vi "Set all to no debugging.vi"() -> ()   [LabVIEW 2013]
doc: "This .vi searches all .vi's in memory and returns a list sorted by the amount memory they are using. This .vi is helpful to find .vis that have stored large amounts of data on the diagram or in the default values."
panel:
  in  "Debug?":bool
  out "total # of .vis":i32=1555
  out "Array":T1(array[cluster])=[{"Boolean"=FALSE, "Boolean 2"=FALSE, "Name"="Quartz MAIN.vi", "Boolean 3"=FALSE}, {"Boolean"=FALSE, "Boolean 2"=FALSE, "Name"="PI Open Interface of one system.vi", "Boolean 3"=FALSE}, {"Boolean"=FALSE, "Boolean 2"=FALSE, "Name"="GCSTranslator DLL Functions.vi", "Boolean 3"=FALSE}, {"Boolean"=FALSE, "Boolean 2"=FALSE, "Name"="HHMI - Zernike GUI.vi", "Boolean 3"=FALSE}, {"Boolean"=FALSE, "Boolean 2"=FALSE, "Name"="Quartz SLM utility.vi", "Boolean 3"=FALSE}, {"Boolean"=FALSE, "Boolean 2"=FALSE, "Name"="HHMI - AO mask definitions.vi", "Boolean 3"=FALSE}, {"Boolean"=FALSE, "Boolean 2"=FALSE, "Name"="Quartz Reviewer.vi", "Boolean 3"=FALSE}, {"Boolean"=FALSE, "Boolean 2"=FALSE, "Name"="C867_Configuration_Setup.vi", "Boolean 3"=FALSE}, {"Boolean"=FALSE, "Boolean 2"=FALSE, "Name"="HHMI - AO Scan Independent mode.vi", "Boolean 3"=FALSE}, {"Boolean"=FALSE, "Boolean 2"=FALSE, "Name"="HHMI - Pick XYlineZ GUI.vi", "Boolean 3"=FALSE}, {"Boolean"=FALSE, "Boolean 2"=FALSE, "Name"="HHMI - Optimize SLM angles and phases simplified inverse.vi", "Boolean 3"=FALSE}, {"Boolean"=FALSE, "Boolean 2"=FALSE, "Name"="HHMI - AO Overlap mode.vi", "Boolean 3"=FALSE}, {"Boolean"=FALSE, "Boolean 2"=FALSE, "Name"="HHMI - AO Scan Masks mode.vi", "Boolean 3"=FALSE}, {"Boolean"=FALSE, "Boolean 2"=FALSE, "Name"="HHMI - SLM Control Module.vi", "Boolean 3"=FALSE}, {"Boolean"=FALSE, "Boolean 2"=FALSE, "Name"="General wait for movement to stop.vi", "Boolean 3"=FALSE}, {"Boolean"=FALSE, "Boolean 2"=FALSE, "Name"="HHMI - Optimize SLM angles and phases for Masks.vi", "Boolean 3"=FALSE}, {"Boolean"=FALSE, "Boolean 2"=FALSE, "Name"="Select DaisyChain device.vi", "Boolean 3"=FALSE}, {"Boolean"=FALSE, "Boolean 2"=FALSE, "Name"="HHMI - AO Scan Inverse mode.vi", "Boolean 3"=FALSE}, {"Boolean"=FALSE, "Boolean 2"=FALSE, "Name"="HHMI - Optimize SLM angles independent montage.vi", "Boolean 3"=FALSE}, {"Boolean"=FALSE, "Boolean 2"=FALSE, "Name"="Select USB device.vi", "Boolean 3"=FALSE}, {"Boolean"=FALSE, "Boolean 2"=FALSE, "Name"="32 bit tiff reader.lvlib:Load Flattened 32bit float Image from Tiff.vi", "Boolean 3"=FALSE}, {"Boolean"=FALSE, "Boolean 2"=FALSE, "Name"="HHMI - Motion GUI.vi", "Boolean 3"=FALSE}, {"Boolean"=FALSE, "Boolean 2"=FALSE, "Name"="HHMI - Align to SLM center calibrate BR image shift Scan module.vi", "Boolean 3"=FALSE}, {"Boolean"=FALSE, "Boolean 2"=FALSE, "Name"="HHMI - Optimize SLM angles simplified inverse.vi", "Boolean 3"=FALSE}, {"Boolean"=FALSE, "Boolean 2"=FALSE, "Name"="HHMI - AO Power Manager.vi", "Boolean 3"=FALSE}, {"Boolean"=FALSE, "Boolean 2"=FALSE, "Name"="HHMI - Optimize SLM phases independent.vi", "Boolean 3"=FALSE}, {"Boolean"=FALSE, "Boolean 2"=FALSE, "Name"="su10x Get Filter Wheel Status.vi", "Boolean 3"=FALSE}, {"Boolean"=FALSE, "Boolean 2"=FALSE, "Name"="PI Receive String.vi", "Boolean 3"=FALSE}, {"Boolean"=FALSE, "Boolean 2"=FALSE, "Name"="HHMI - Optimize SLM angles Masks.vi", "Boolean 3"=FALSE}, {"Boolean"=FALSE, "Boolean 2"=FALSE, "Name"="HHMI - Optimize SLM phase of 1 mask.vi", "Boolean 3"=FALSE}, {"Boolean"=FALSE, "Boolean 2"=FALSE, "Name"="HHMI - Align to each SLM subregion Scan module.vi", "Boolean 3"=FALSE}, {"Boolean"=FALSE, "Boolean 2"=FALSE, "Name"="HHMI - Optimize SLM phase of 1 subregion independent.vi", "Boolean 3"=FALSE}, {"Boolean"=FALSE, "Boolean 2"=FALSE, "Name"="HHMI - PI laser motion module.vi", "Boolean 3"=FALSE}, {"Boolean"=FALSE, "Boolean 2"=FALSE, "Name"="HHMI - Optimize SLM angles Overlap.vi", "Boolean 3"=FALSE}, {"Boolean"=FALSE, "Boolean 2"=FALSE, "Name"="Adjust Laser positioner Calibration GUI.vi", "Boolean 3"=FALSE}, {"Boolean"=FALSE, "Boolean 2"=FALSE, "Name"="HHMI - Optimize SLM angles independent.vi", "Boolean 3"=FALSE}, {"Boolean"=FALSE, "Boolean 2"=FALSE, "Name"="HHMI - Optimize SLM phase of 1 subsubregion inverse.vi", "Boolean 3"=FALSE}, {"Boolean"=FALSE, "Boolean 2"=FALSE, "Name"="HHMI - Optimize SLM angles and phases for Overlap.vi", "Boolean 3"=FALSE}, {"Boolean"=FALSE, "Boolean 2"=FALSE, "Name"="Assign values from string to axes.vi", "Boolean 3"=FALSE}, {"Boolean"=FALSE, "Boolean 2"=FALSE, "Name"="HHMI - Subregion On Scan module.vi", "Boolean 3"=FALSE}, {"Boolean"=FALSE, "Boolean 2"=FALSE, "Name"="HHMI - Working images - create and keep reference.vi", "Boolean 3"=FALSE}, {"Boolean"=FALSE, "Boolean 2"=FALSE, "Name"="HHMI - Joystick control loop.vi", "Boolean 3"=FALSE}, {"Boolean"=FALSE, "Boolean 2"=FALSE, "Name"="HHMI - Subregion Off Scan module.vi", "Boolean 3"=FALSE}, {"Boolean"=FALSE, "Boolean 2"=FALSE, "Name"="HHMI - Calc Single X Line Ramp.vi", "Boolean 3"=FALSE}, {"Boolean"=FALSE, "Boolean 2"=FALSE, "Name"="HHMI - Linescan Scan module.vi", "Boolean 3"=FALSE}, {"Boolean"=FALSE, "Boolean 2"=FALSE, "Name"="HHMI - Analysis Table module.vi", "Boolean 3"=FALSE}, {"Boolean"=FALSE, "Boolean 2"=FALSE, "Name"="HHMI - Retrieve All Settings from globals.vi", "Boolean 3"=FALSE}, {"Boolean"=FALSE, "Boolean 2"=FALSE, "Name"="HHMI - Center laser along one axis module.vi", "Boolean 3"=FALSE}, {"Boolean"=FALSE, "Boolean 2"=FALSE, "Name"="HHMI - Center laser to on subregions module.vi", "Boolean 3"=FALSE}, {"Boolean"=FALSE, "Boolean 2"=FALSE, "Name"="SO Beam expander.lvlib:SO - BE Controller used now for calibration only.vi", "Boolean 3"=FALSE}, {"Boolean"=FALSE, "Boolean 2"=FALSE, "Name"="HHMI - Beam size control module.vi", "Boolean 3"=FALSE}, {"Boolean"=FALSE, "Boolean 2"=FALSE, "Name"="HHMI - Z Stack Scan module.vi", "Boolean 3"=FALSE}, {"Boolean"=FALSE, "Boolean 2"=FALSE, "Name"="HHMI - Optimize SLM phases for Masks.vi", "Boolean 3"=FALSE}, {"Boolean"=FALSE, "Boolean 2"=FALSE, "Name"="HHMI - Global ramp generate subregion offsets.vi", "Boolean 3"=FALSE}, {"Boolean"=FALSE, "Boolean 2"=FALSE, "Name"="HHMI - Locate blob.vi", "Boolean 3"=FALSE}, {"Boolean"=FALSE, "Boolean 2"=FALSE, "Name"="PI Send String.vi", "Boolean 3"=FALSE}, {"Boolean"=FALSE, "Boolean 2"=FALSE, "Name"="HHMI - Increase OL subregion resolution and extend planes to border.vi", "Boolean 3"=FALSE}, {"Boolean"=FALSE, "Boolean 2"=FALSE, "Name"="HHMI - PI beam reducer module.vi", "Boolean 3"=FALSE}, {"Boolean"=FALSE, "Boolean 2"=FALSE, "Name"="HHMI - Align to SLM active area Scan module.vi", "Boolean 3"=FALSE}, {"Boolean"=FALSE, "Boolean 2"=FALSE, "Name"="HHMI - Wait for scan to finish.vi", "Boolean 3"=FALSE}, {"Boolean"=FALSE, "Boolean 2"=FALSE, "Name"="HHMI - Configure for scan.vi", "Boolean 3"=FALSE}, {"Boolean"=FALSE, "Boolean 2"=FALSE, "Name"="HHMI - Optimize SLM phase simplified inverse.vi", "Boolean 3"=FALSE}, {"Boolean"=FALSE, "Boolean 2"=FALSE, "Name"="Adjust BR Calibration GUI.vi", "Boolean 3"=FALSE}, {"Boolean"=FALSE, "Boolean 2"=FALSE, "Name"="HHMI - Adjust power up or down based on current signal.vi", "Boolean 3"=FALSE}, {"Boolean"=FALSE, "Boolean 2"=FALSE, "Name"="Assign booleans from string to axes.vi", "Boolean 3"=FALSE}, {"Boolean"=FALSE, "Boolean 2"=FALSE, "Name"="HHMI - Generate Waveform.vi", "Boolean 3"=FALSE}, {"Boolean"=FALSE, "Boolean 2"=FALSE, "Name"="HHMI - Stage 1 optimized beamlet settings storage global.vi", "Boolean 3"=FALSE}, {"Boolean"=FALSE, "Boolean 2"=FALSE, "Name"="HHMI - Optimized Beamlet settings storage global.vi", "Boolean 3"=FALSE}, {"Boolean"=FALSE, "Boolean 2"=FALSE, "Name"="Alignment GUI.vi", "Boolean 3"=FALSE}, {"Boolean"=FALSE, "Boolean 2"=FALSE, "Name"="HHMI - Scan.vi", "Boolean 3"=FALSE}, {"Boolean"=FALSE, "Boolean 2"=FALSE, "Name"="HHMI - Convert one channel to Pixels.vi", "Boolean 3"=FALSE}, {"Boolean"=FALSE, "Boolean 2"=FALSE, "Name"="HHMI - Select a coordinate GUI.vi", "Boolean 3"=FALSE}, {"Boolean"=FALSE, "Boolean 2"=FALSE, "Name"="HHMI - Magnify and Center waveform on phase signal area.vi", "Boolean 3"=FALSE}, {"Boolean"=FALSE, "Boolean 2"=FALSE, "Name"="HHMI - Shift waveforms by galvo delay.vi", "Boolean 3"=FALSE}, {"Boolean"=FALSE, "Boolean 2"=FALSE, "Name"="HHMI - Generate 1 Frame Sine.vi", "Boolean 3"=FALSE}, {"Boolean"=FALSE, "Boolean 2"=FALSE, "Name"="HHMI - Generate 1 Frame Ramp.vi", "Boolean 3"=FALSE}, {"Boolean"=FALSE, "Boolean 2"=FALSE, "Name"="HHMI - XY Galvo control module.vi", "Boolean 3"=FALSE}, {"Boolean"=FALSE, "Boolean 2"=FALSE, "Name"="HHMI - Generate subdivided subsubregions.vi", "Boolean 3"=FALSE}, {"Boolean"=FALSE, "Boolean 2"=FALSE, "Name"="HHMI - Lev Mar.vi", "Boolean 3"=FALSE}, {"Boolean"=FALSE, "Boolean 2"=FALSE, "Name"="HHMI - AO Dev3 control module.vi", "Boolean 3"=FALSE}, {"Boolean"=FALSE, "Boolean 2"=FALSE, "Name"="HHMI - Z Pockel control module.vi", "Boolean 3"=FALSE}, {"Boolean"=FALSE, "Boolean 2"=FALSE, "Name"="HHMI - XY Continuous Scan module.vi", "Boolean 3"=FALSE}, {"Boolean"=FALSE, "Boolean 2"=FALSE, "Name"="HHMI - XY Single Scan module.vi", "Boolean 3"=FALSE}, {"Boolean"=FALSE, "Boolean 2"=FALSE, "Name"="HHMI - Dynamically launch Pick XYlineZ GUI.vi", "Boolean 3"=FALSE}, {"Boolean"=FALSE, "Boolean 2"=FALSE, "Name"="HHMI - Initialize for AO Overlap Scan.vi", "Boolean 3"=FALSE}, {"Boolean"=FALSE, "Boolean 2"=FALSE, "Name"="HHMI - Is a new Background scan needed for this waveform config.vi", "Boolean 3"=FALSE}, {"Boolean"=FALSE, "Boolean 2"=FALSE, "Name"="HHMI - Generate 1 Line Sine.vi", "Boolean 3"=FALSE}, {"Boolean"=FALSE, "Boolean 2"=FALSE, "Name"="HHMI - Calc Single Frame Ramp Waveform.vi", "Boolean 3"=FALSE}, {"Boolean"=FALSE, "Boolean 2"=FALSE, "Name"="HHMI - Optimized Beamlet settings for Pre-Angle and Pre-Phase storage global.vi", "Boolean 3"=FALSE}, {"Boolean"=FALSE, "Boolean 2"=FALSE, "Name"="HHMI - Beam reducer in scan and store COM as ref.vi", "Boolean 3"=FALSE}, {"Boolean"=FALSE, "Boolean 2"=FALSE, "Name"="HHMI - ReadWrite Analysis Info.vi", "Boolean 3"=FALSE}, {"Boolean"=FALSE, "Boolean 2"=FALSE, "Name"="HHMI - Z stack settings functional global.vi", "Boolean 3"=FALSE}, {"Boolean"=FALSE, "Boolean 2"=FALSE, "Name"="HHMI - AO Scan wrapper.vi", "Boolean 3"=FALSE}, {"Boolean"=FALSE, "Boolean 2"=FALSE, "Name"="HHMI - Generate 1 Line Ramp.vi", "Boolean 3"=FALSE}, {"Boolean"=FALSE, "Boolean 2"=FALSE, "Name"="HHMI - Turn on one subregion, one mask, or one overlap region on_Also scan if no BR is used.vi", "Boolean 3"=FALSE}, {"Boolean"=FALSE, "Boolean 2"=FALSE, "Name"="HHMI - Fit Phase with Zernike modes using nonlinear fit 1 iteration.vi", "Boolean 3"=FALSE}, {"Boolean"=FALSE, "Boolean 2"=FALSE, "Name"="HHMI - PMT and Integrator Acquisition control module.vi", "Boolean 3"=FALSE}, {"Boolean"=FALSE, "Boolean 2"=FALSE, "Name"="su10x Get Filter Wheel Configuration.vi", "Boolean 3"=FALSE}, {"Boolean"=FALSE, "Boolean 2"=FALSE, "Name"="HHMI - Initialize for Independent AO Scan.vi", "Boolean 3"=FALSE}, {"Boolean"=FALSE, "Boolean 2"=FALSE, "Name"="HHMI - Image Correlation module.vi", "Boolean 3"=FALSE}, {"Boolean"=FALSE, "Boolean 2"=FALSE, "Name"="Joystick controller.vi", "Boolean 3"=FALSE}, {"Boolean"=FALSE, "Boolean 2"=FALSE, "Name"="HHMI - Extend 2D subregion array with one element border.vi", "Boolean 3"=FALSE}, {"Boolean"=FALSE, "Boolean 2"=FALSE, "Name"="HHMI - Initialize for AO Mask Scan.vi", "Boolean 3"=FALSE}, {"Boolean"=FALSE, "Boolean 2"=FALSE, "Name"="HHMI - Background image storage module.vi", "Boolean 3"=FALSE}, {"Boolean"=FALSE, "Boolean 2"=FALSE, "Name"="Cut out additional spaces.vi", "Boolean 3"=FALSE}, {"Boolean"=FALSE, "Boolean 2"=FALSE, "Name"="HHMI - Unwrap Phase.vi", "Boolean 3"=FALSE}, {"Boolean"=FALSE, "Boolean 2"=FALSE, "Name"="HHMI - Send image to logger loop.vi", "Boolean 3"=FALSE}, {"Boolean"=FALSE, "Boolean 2"=FALSE, "Name"="HHMI - Calibrated XY image shift due to beam expander functional global.vi", "Boolean 3"=FALSE}, {"Boolean"=FALSE, "Boolean 2"=FALSE, "Name"="HHMI - Phase Signal storage global.vi", "Boolean 3"=FALSE}, {"Boolean"=FALSE, "Boolean 2"=FALSE, "Name"="HHMI - Convert between Settings cluster and flattenned string.vi", "Boolean 3"=FALSE}, {"Boolean"=FALSE, "Boolean 2"=FALSE, "Name"="HHMI - Optimize SLM phases via wavefront reconstruction.vi", "Boolean 3"=FALSE}, {"Boolean"=FALSE, "Boolean 2"=FALSE, "Name"="HHMI - Goto XYZ.vi", "Boolean 3"=FALSE}, {"Boolean"=FALSE, "Boolean 2"=FALSE, "Name"="HHMI - Cal Zernike Mode.vi", "Boolean 3"=FALSE}, {"Boolean"=FALSE, "Boolean 2"=FALSE, "Name"="Adjust waveform for montage.vi", "Boolean 3"=FALSE}, {"Boolean"=FALSE, "Boolean 2"=FALSE, "Name"="HHMI - Generate Waveform Sine.vi", "Boolean 3"=FALSE}, {"Boolean"=FALSE, "Boolean 2"=FALSE, "Name"="HHMI - Generate Waveform Ramp.vi", "Boolean 3"=FALSE}, {"Boolean"=FALSE, "Boolean 2"=FALSE, "Name"="HHMI - Process image for COM calc.vi", "Boolean 3"=FALSE}, {"Boolean"=FALSE, "Boolean 2"=FALSE, "Name"="HHMI - XY Position and Electrode Acquisition control module.vi", "Boolean 3"=FALSE}, {"Boolean"=FALSE, "Boolean 2"=FALSE, "Name"="Interpolate 2D uneven arrays full calc.vi", "Boolean 3"=FALSE}, {"Boolean"=FALSE, "Boolean 2"=FALSE, "Name"="HHMI - Z elevator motion module.vi", "Boolean 3"=FALSE}, {"Boolean"=FALSE, "Boolean 2"=FALSE, "Name"="HHMI - Scale Image.vi", "Boolean 3"=FALSE}, {"Boolean"=FALSE, "Boolean 2"=FALSE, "Name"="HHMI - Alignment Scan wrapper.vi", "Boolean 3"=FALSE}, {"Boolean"=FALSE, "Boolean 2"=FALSE, "Name"="HHMI - Pockel PD Acquisition control module.vi", "Boolean 3"=FALSE}, {"Boolean"=FALSE, "Boolean 2"=FALSE, "Name"="HHMI - Take Ref scan or scans with one mask on.vi", "Boolean 3"=FALSE}, {"Boolean"=FALSE, "Boolean 2"=FALSE, "Name"="HHMI - Take Ref scan or scans with one overlap region on.vi", "Boolean 3"=FALSE}, {"Boolean"=FALSE, "Boolean 2"=FALSE, "Name"="HHMI - XY table motion module.vi", "Boolean 3"=FALSE}, {"Boolean"=FALSE, "Boolean 2"=FALSE, "Name"="HHMI - Center waveform config at COM coords.vi", "Boolean 3"=FALSE}, {"Boolean"=FALSE, "Boolean 2"=FALSE, "Name"="HHMI - Autoset power functional global.vi", "Boolean 3"=FALSE}, {"Boolean"=FALSE, "Boolean 2"=FALSE, "Name"="HHMI - Fit and Store mask as optimized if improved.vi", "Boolean 3"=FALSE}, {"Boolean"=FALSE, "Boolean 2"=FALSE, "Name"="HHMI - Lookup table for Stage mm to SLM mm functional global.vi", "Boolean 3"=FALSE}, {"Boolean"=FALSE, "Boolean 2"=FALSE, "Name"="Wait for axes to stop.vi", "Boolean 3"=FALSE}, {"Boolean"=FALSE, "Boolean 2"=FALSE, "Name"="HHMI - Scan centered at the COM or Image Correlation user selection.vi", "Boolean 3"=FALSE}, {"Boolean"=FALSE, "Boolean 2"=FALSE, "Name"="HHMI - Subregion Scan wrapper.vi", "Boolean 3"=FALSE}, {"Boolean"=FALSE, "Boolean 2"=FALSE, "Name"="HHMI - Image ROI to XY Parameters.vi", "Boolean 3"=FALSE}, {"Boolean"=FALSE, "Boolean 2"=FALSE, "Name"="HHMI - Extend subregion plane to neighboring subregions.vi", "Boolean 3"=FALSE}, {"Boolean"=FALSE, "Boolean 2"=FALSE, "Name"="HHMI - Check and correct Fast axis params.vi", "Boolean 3"=FALSE}, {"Boolean"=FALSE, "Boolean 2"=FALSE, "Name"="HHMI - Subdivide optimized SLM image.vi", "Boolean 3"=FALSE}, {"Boolean"=FALSE, "Boolean 2"=FALSE, "Name"="HHMI - Prepare for alignment to all SLM regions.vi", "Boolean 3"=FALSE}, {"Boolean"=FALSE, "Boolean 2"=FALSE, "Name"="HHMI - Simulate Scan.vi", "Boolean 3"=FALSE}, {"Boolean"=FALSE, "Boolean 2"=FALSE, "Name"="Wait for hexapod system axes to stop.vi", "Boolean 3"=FALSE}, {"Boolean"=FALSE, "Boolean 2"=FALSE, "Name"="HHMI - Laser Power storage functional global.vi", "Boolean 3"=FALSE}, {"Boolean"=FALSE, "Boolean 2"=FALSE, "Name"="HHMI - All on scan for Masks to accept or reject current mask set.vi", "Boolean 3"=FALSE}, {"Boolean"=FALSE, "Boolean 2"=FALSE, "Name"="HHMI - Calc Single Frame Sine Waveform.vi", "Boolean 3"=FALSE}, {"Boolean"=FALSE, "Boolean 2"=FALSE, "Name"="HHMI - Increase Power Time or Averages to get more Signal.vi", "Boolean 3"=FALSE}, {"Boolean"=FALSE, "Boolean 2"=FALSE, "Name"="HHMI - Calc X Sine Waveform.vi", "Boolean 3"=FALSE}, {"Boolean"=FALSE, "Boolean 2"=FALSE, "Name"="SO Beam expander.lvlib:Gen_7I60_IO.vi", "Boolean 3"=FALSE}, {"Boolean"=FALSE, "Boolean 2"=FALSE, "Name"="HHMI - Generate pattern.vi", "Boolean 3"=FALSE}, {"Boolean"=FALSE, "Boolean 2"=FALSE, "Name"="HHMI - Scan state information to Strings.vi", "Boolean 3"=FALSE}, {"Boolean"=FALSE, "Boolean 2"=FALSE, "Name"="HHMI - Overlap settings to number of duplicate rows and columns.vi", "Boolean 3"=FALSE}, {"Boolean"=FALSE, "Boolean 2"=FALSE, "Name"="HHMI - Background Module.vi", "Boolean 3"=FALSE}, {"Boolean"=FALSE, "Boolean 2"=FALSE, "Name"="HHMI - Overlap wavefront reconstruction storage global.vi", "Boolean 3"=FALSE}, {"Boolean"=FALSE, "Boolean 2"=FALSE, "Name"="Increase image size for montage.vi", "Boolean 3"=FALSE}, {"Boolean"=FALSE, "Boolean 2"=FALSE, "Name"="HHMI - Number of extra counts needed for galvo iteria shift.vi", "Boolean 3"=FALSE}, {"Boolean"=FALSE, "Boolean 2"=FALSE, "Name"="HHMI - SLM Sizes.vi", "Boolean 3"=FALSE}, {"Boolean"=FALSE, "Boolean 2"=FALSE, "Name"="HHMI - Add Signal overlay to image.vi", "Boolean 3"=FALSE}, {"Boolean"=FALSE, "Boolean 2"=FALSE, "Name"="HHMI - Add COM overlay to image.vi", "Boolean 3"=FALSE}, {"Boolean"=FALSE, "Boolean 2"=FALSE, "Name"="SO Beam expander.lvlib:Seek_Home.vi", "Boolean 3"=FALSE}, {"Boolean"=FALSE, "Boolean 2"=FALSE, "Name"="HHMI - Read or write SLM settings.vi", "Boolean 3"=FALSE}, {"Boolean"=FALSE, "Boolean 2"=FALSE, "Name"="HHMI - Check AO rate.vi", "Boolean 3"=FALSE}, {"Boolean"=FALSE, "Boolean 2"=FALSE, "Name"="HHMI - Find Max laser power.vi", "Boolean 3"=FALSE}, {"Boolean"=FALSE, "Boolean 2"=FALSE, "Name"="HHMI - Lock image size.vi", "Boolean 3"=FALSE}, {"Boolean"=FALSE, "Boolean 2"=FALSE, "Name"="Interloop message handler.vi", "Boolean 3"=FALSE}, {"Boolean"=FALSE, "Boolean 2"=FALSE, "Name"="HHMI - Add phase info to table.vi", "Boolean 3"=FALSE}, {"Boolean"=FALSE, "Boolean 2"=FALSE, "Name"="HHMI - Generate Slow axis array for sine.vi", "Boolean 3"=FALSE}, {"Boolean"=FALSE, "Boolean 2"=FALSE, "Name"="HHMI - Pixel Clock control module.vi", "Boolean 3"=FALSE}, {"Boolean"=FALSE, "Boolean 2"=FALSE, "Name"="SO Beam expander.lvlib:Tweak.vi", "Boolean 3"=FALSE}, {"Boolean"=FALSE, "Boolean 2"=FALSE, "Name"="HHMI - Place subregion array into display array.vi", "Boolean 3"=FALSE}, {"Boolean"=FALSE, "Boolean 2"=FALSE, "Name"="HHMI - Image buffer logger.vi", "Boolean 3"=FALSE}, {"Boolean"=FALSE, "Boolean 2"=FALSE, "Name"="SAI?.vi", "Boolean 3"=FALSE}, {"Boolean"=FALSE, "Boolean 2"=FALSE, "Name"="HHMI - Beam reducer shift image in waveform.vi", "Boolean 3"=FALSE}, {"Boolean"=FALSE, "Boolean 2"=FALSE, "Name"="HHMI - Crop SLM pixels to subregions.vi", "Boolean 3"=FALSE}, {"Boolean"=FALSE, "Boolean 2"=FALSE, "Name"="SO Beam expander.lvlib:Read Config INI.vi", "Boolean 3"=FALSE}, {"Boolean"=FALSE, "Boolean 2"=FALSE, "Name"="HHMI - Check Coordinates.vi", "Boolean 3"=FALSE}, {"Boolean"=FALSE, "Boolean 2"=FALSE, "Name"="HHMI - Read write Axis cluster from Waveform.vi", "Boolean 3"=FALSE}, {"Boolean"=FALSE, "Boolean 2"=FALSE, "Name"="HHMI - AO move Beam reducer.vi", "Boolean 3"=FALSE}, {"Boolean"=FALSE, "Boolean 2"=FALSE, "Name"="HHMI - Displacement Data storage global.vi", "Boolean 3"=FALSE}, {"Boolean"=FALSE, "Boolean 2"=FALSE, "Name"="Is DaisyChain open.vi", "Boolean 3"=FALSE}, {"Boolean"=FALSE, "Boolean 2"=FALSE, "Name"="HHMI - Generate Zernike Bar graph.vi", "Boolean 3"=FALSE}, {"Boolean"=FALSE, "Boolean 2"=FALSE, "Name"="HHMI - Calc optimized offset of multiple subregions using neighboring subregions.vi", "Boolean 3"=FALSE}, {"Boolean"=FALSE, "Boolean 2"=FALSE, "Name"="HHMI - Set Reducer and waveform.vi", "Boolean 3"=FALSE}, {"Boolean"=FALSE, "Boolean 2"=FALSE, "Name"="HHMI - Calculate Signal.vi", "Boolean 3"=FALSE}, {"Boolean"=FALSE, "Boolean 2"=FALSE, "Name"="HHMI - Integrator Pulse control module.vi", "Boolean 3"=FALSE}, {"Boolean"=FALSE, "Boolean 2"=FALSE, "Name"="HHMI - Store current settings as initial speed and power.vi", "Boolean 3"=FALSE}, {"Boolean"=FALSE, "Boolean 2"=FALSE, "Name"="HHMI - Overlap settings to number of rows and columns.vi", "Boolean 3"=FALSE}, {"Boolean"=FALSE, "Boolean 2"=FALSE, "Name"="HHMI - Load SLM image from file.vi", "Boolean 3"=FALSE}, {"Boolean"=FALSE, "Boolean 2"=FALSE, "Name"="Interpolate 2D uneven arrays linear fit row by row.vi", "Boolean 3"=FALSE}, {"Boolean"=FALSE, "Boolean 2"=FALSE, "Name"="HHMI - Reset Waveform Configuration to initial power and scan speed.vi", "Boolean 3"=FALSE}, {"Boolean"=FALSE, "Boolean 2"=FALSE, "Name"="HHMI - Is SLM setup for masks.vi", "Boolean 3"=FALSE}, {"Boolean"=FALSE, "Boolean 2"=FALSE, "Name"="HHMI - Generate subregion block from subregion settings.vi", "Boolean 3"=FALSE}, {"Boolean"=FALSE, "Boolean 2"=FALSE, "Name"="HHMI - Set power for 1 mask.vi", "Boolean 3"=FALSE}, {"Boolean"=FALSE, "Boolean 2"=FALSE, "Name"="HHMI - Load Image and Settings from File.vi", "Boolean 3"=FALSE}, {"Boolean"=FALSE, "Boolean 2"=FALSE, "Name"="SO Beam expander.lvlib:Intialize Serial Port.vi", "Boolean 3"=FALSE}, {"Boolean"=FALSE, "Boolean 2"=FALSE, "Name"="HHMI - Prepare for alignment to active SLM regions.vi", "Boolean 3"=FALSE}, {"Boolean"=FALSE, "Boolean 2"=FALSE, "Name"="HHMI - Unwrap Phase down each row of subregions.vi", "Boolean 3"=FALSE}, {"Boolean"=FALSE, "Boolean 2"=FALSE, "Name"="HHMI - Unwrap Phase down each column of subregions.vi", "Boolean 3"=FALSE}, {"Boolean"=FALSE, "Boolean 2"=FALSE, "Name"="HHMI - AO set beam size.vi", "Boolean 3"=FALSE}, {"Boolean"=FALSE, "Boolean 2"=FALSE, "Name"="HHMI - Subregion powers and dwell time functional global.vi", "Boolean 3"=FALSE}, {"Boolean"=FALSE, "Boolean 2"=FALSE, "Name"="HHMI - Digital input output DC control module.vi", "Boolean 3"=FALSE}, {"Boolean"=FALSE, "Boolean 2"=FALSE, "Name"="HHMI - Find ROI.vi", "Boolean 3"=FALSE}, {"Boolean"=FALSE, "Boolean 2"=FALSE, "Name"="HHMI - Sutter filter wheel module.vi", "Boolean 3"=FALSE}, {"Boolean"=FALSE, "Boolean 2"=FALSE, "Name"="Initialize Global1.vi", "Boolean 3"=FALSE}, {"Boolean"=FALSE, "Boolean 2"=FALSE, "Name"="HHMI - Reduce Power to prevent saturation.vi", "Boolean 3"=FALSE}, {"Boolean"=FALSE, "Boolean 2"=FALSE, "Name"="HHMI - Signal vs Motion storage global.vi", "Boolean 3"=FALSE}, {"Boolean"=FALSE, "Boolean 2"=FALSE, "Name"="HHMI - Line Profile.vi", "Boolean 3"=FALSE}, {"Boolean"=FALSE, "Boolean 2"=FALSE, "Name"="su10x Initialize.vi", "Boolean 3"=FALSE}, {"Boolean"=FALSE, "Boolean 2"=FALSE, "Name"="HHMI - Add File image pixels to SLM subregion.vi", "Boolean 3"=FALSE}, {"Boolean"=FALSE, "Boolean 2"=FALSE, "Name"="HHMI - SLM pixels to Laser mm functional global.vi", "Boolean 3"=FALSE}, {"Boolean"=FALSE, "Boolean 2"=FALSE, "Name"="HHMI - Set the previous power and dwell time for a subregion.vi", "Boolean 3"=FALSE}, {"Boolean"=FALSE, "Boolean 2"=FALSE, "Name"="SO Beam expander.lvlib:Move Both.vi", "Boolean 3"=FALSE}, {"Boolean"=FALSE, "Boolean 2"=FALSE, "Name"="HHMI - Move Laser on SLM.vi", "Boolean 3"=FALSE}, {"Boolean"=FALSE, "Boolean 2"=FALSE, "Name"="HHMI - Set power for 1 overlap region.vi", "Boolean 3"=FALSE}, {"Boolean"=FALSE, "Boolean 2"=FALSE, "Name"="HHMI - Running Center of mass.vi", "Boolean 3"=FALSE}, {"Boolean"=FALSE, "Boolean 2"=FALSE, "Name"="3D Polynomial Fit.vi", "Boolean 3"=FALSE}, {"Boolean"=FALSE, "Boolean 2"=FALSE, "Name"="HHMI - Manually select coordinates if in correct mode.vi", "Boolean 3"=FALSE}, {"Boolean"=FALSE, "Boolean 2"=FALSE, "Name"="HHMI - Adjust subregion resolution.vi", "Boolean 3"=FALSE}, {"Boolean"=FALSE, "Boolean 2"=FALSE, "Name"="HHMI - Compute Image Shift using Image Correlation.vi", "Boolean 3"=FALSE}, {"Boolean"=FALSE, "Boolean 2"=FALSE, "Name"="HHMI - Prepare subregion to be placed in centered SLM image.vi", "Boolean 3"=FALSE}, {"Boolean"=FALSE, "Boolean 2"=FALSE, "Name"="HHMI - Zernike Image fit.vi", "Boolean 3"=FALSE}, {"Boolean"=FALSE, "Boolean 2"=FALSE, "Name"="HHMI - Add image to write to disk buffer.vi", "Boolean 3"=FALSE}, {"Boolean"=FALSE, "Boolean 2"=FALSE, "Name"="Simple Image load.vi", "Boolean 3"=FALSE}, {"Boolean"=FALSE, "Boolean 2"=FALSE, "Name"="HHMI - Scan speed storage functional global.vi", "Boolean 3"=FALSE}, {"Boolean"=FALSE, "Boolean 2"=FALSE, "Name"="Spiral indices.vi", "Boolean 3"=FALSE}, {"Boolean"=FALSE, "Boolean 2"=FALSE, "Name"="HHMI - Unwrap Phase spiraling through subregions and use neighbors.vi", "Boolean 3"=FALSE}, {"Boolean"=FALSE, "Boolean 2"=FALSE, "Name"="Interpolate 2D uneven arrays row by row.vi", "Boolean 3"=FALSE}, {"Boolean"=FALSE, "Boolean 2"=FALSE, "Name"="HHMI - Zernike Mode calculation buffer.vi", "Boolean 3"=FALSE}, {"Boolean"=FALSE, "Boolean 2"=FALSE, "Name"="HHMI - Add data to image buffer.vi", "Boolean 3"=FALSE}, {"Boolean"=FALSE, "Boolean 2"=FALSE, "Name"="HHMI - Generate subregion and add to SLM image.vi", "Boolean 3"=FALSE}, {"Boolean"=FALSE, "Boolean 2"=FALSE, "Name"="HHMI - Set power for 1 subregion.vi", "Boolean 3"=FALSE}, {"Boolean"=FALSE, "Boolean 2"=FALSE, "Name"="HHMI - Fit Phase with Zernike modes using nonlinear fit.vi", "Boolean 3"=FALSE}, {"Boolean"=FALSE, "Boolean 2"=FALSE, "Name"="HHMI - Find border pixel arrays from array.vi", "Boolean 3"=FALSE}, {"Boolean"=FALSE, "Boolean 2"=FALSE, "Name"="HHMI - Generate Slow axis array for ramp.vi", "Boolean 3"=FALSE}, {"Boolean"=FALSE, "Boolean 2"=FALSE, "Name"="HHMI - Image Log functional global.vi", "Boolean 3"=FALSE}, {"Boolean"=FALSE, "Boolean 2"=FALSE, "Name"="HHMI - Background Manager.vi", "Boolean 3"=FALSE}, {"Boolean"=FALSE, "Boolean 2"=FALSE, "Name"="HHMI - Waveform Config functional global.vi", "Boolean 3"=FALSE}, {"Boolean"=FALSE, "Boolean 2"=FALSE, "Name"="HHMI - Fit Laser Position Calibration to plane.vi", "Boolean 3"=FALSE}, {"Boolean"=FALSE, "Boolean 2"=FALSE, "Name"="HHMI - Find beamlet shift.vi", "Boolean 3"=FALSE}, {"Boolean"=FALSE, "Boolean 2"=FALSE, "Name"="HHMI - Global ramp generate shifted subregions.vi", "Boolean 3"=FALSE}, {"Boolean"=FALSE, "Boolean 2"=FALSE, "Name"="HHMI - Store analysis channel to montage buffer.vi", "Boolean 3"=FALSE}, {"Boolean"=FALSE, "Boolean 2"=FALSE, "Name"="HHMI - Set SLM for current overlap region.vi", "Boolean 3"=FALSE}, {"Boolean"=FALSE, "Boolean 2"=FALSE, "Name"="Generate User Palette.vi", "Boolean 3"=FALSE}, {"Boolean"=FALSE, "Boolean 2"=FALSE, "Name"="PI VISA Receive Characters.vi", "Boolean 3"=FALSE}, {"Boolean"=FALSE, "Boolean 2"=FALSE, "Name"="HHMI - Duplicate subregion.vi", "Boolean 3"=FALSE}, {"Boolean"=FALSE, "Boolean 2"=FALSE, "Name"="HHMI - Check and correct Slow axis params.vi", "Boolean 3"=FALSE}, {"Boolean"=FALSE, "Boolean 2"=FALSE, "Name"="HHMI - Determine File Type.vi", "Boolean 3"=FALSE}, {"Boolean"=FALSE, "Boolean 2"=FALSE, "Name"="HHMI - Fit and Store independent as optimized.vi", "Boolean 3"=FALSE}, {"Boolean"=FALSE, "Boolean 2"=FALSE, "Name"="HHMI - Global ramp.vi", "Boolean 3"=FALSE}, {"Boolean"=FALSE, "Boolean 2"=FALSE, "Name"="HHMI - AO mask subregions.vi", "Boolean 3"=FALSE}, {"Boolean"=FALSE, "Boolean 2"=FALSE, "Name"="HHMI - Initialize SLM for AO overlap scan.vi", "Boolean 3"=FALSE}, {"Boolean"=FALSE, "Boolean 2"=FALSE, "Name"="Determine Files to Zip.vi", "Boolean 3"=FALSE}, {"Boolean"=FALSE, "Boolean 2"=FALSE, "Name"="32 bit tiff reader.lvlib:Get Tag Value.vi", "Boolean 3"=FALSE}, {"Boolean"=FALSE, "Boolean 2"=FALSE, "Name"="Close connection if open.vi", "Boolean 3"=FALSE}, {"Boolean"=FALSE, "Boolean 2"=FALSE, "Name"="Set RON and return RON status.vi", "Boolean 3"=FALSE}, {"Boolean"=FALSE, "Boolean 2"=FALSE, "Name"="HHMI - Unwrap Phases for each subregion individually.vi", "Boolean 3"=FALSE}, {"Boolean"=FALSE, "Boolean 2"=FALSE, "Name"="HHMI - Acquire one image.vi", "Boolean 3"=FALSE}, {"Boolean"=FALSE, "Boolean 2"=FALSE, "Name"="HHMI - Convert SLM mm to stage coords via lookup table.vi", "Boolean 3"=FALSE}, {"Boolean"=FALSE, "Boolean 2"=FALSE, "Name"="HHMI - Crop SLM image to subregions (return pixels).vi", "Boolean 3"=FALSE}, {"Boolean"=FALSE, "Boolean 2"=FALSE, "Name"="HHMI - Calculate Beamlet Shift Settings.vi", "Boolean 3"=FALSE}, {"Boolean"=FALSE, "Boolean 2"=FALSE, "Name"="SO Beam expander.lvlib:HHMI - SO Beam Expander Module.vi", "Boolean 3"=FALSE}, {"Boolean"=FALSE, "Boolean 2"=FALSE, "Name"="Get lines from string.vi", "Boolean 3"=FALSE}, {"Boolean"=FALSE, "Boolean 2"=FALSE, "Name"="HHMI - Turn off half of the subregions.vi", "Boolean 3"=FALSE}, {"Boolean"=FALSE, "Boolean 2"=FALSE, "Name"="HHMI - Create SLM Image Array.vi", "Boolean 3"=FALSE}, {"Boolean"=FALSE, "Boolean 2"=FALSE, "Name"="HHMI - Correct Z parameters if not XYlineZ.vi", "Boolean 3"=FALSE}, {"Boolean"=FALSE, "Boolean 2"=FALSE, "Name"="HHMI - Pixel Profile.vi", "Boolean 3"=FALSE}, {"Boolean"=FALSE, "Boolean 2"=FALSE, "Name"="HHMI - Mask for COM calc.vi", "Boolean 3"=FALSE}, {"Boolean"=FALSE, "Boolean 2"=FALSE, "Name"="HHMI - Unwrap Phase down the columns of pixels of a single subregion.vi", "Boolean 3"=FALSE}, {"Boolean"=FALSE, "Boolean 2"=FALSE, "Name"="HHMI - Zernike user settings.vi", "Boolean 3"=FALSE}, {"Boolean"=FALSE, "Boolean 2"=FALSE, "Name"="HHMI - Close all motors.vi", "Boolean 3"=FALSE}, {"Boolean"=FALSE, "Boolean 2"=FALSE, "Name"="HHMI - Remove borders.vi", "Boolean 3"=FALSE}, {"Boolean"=FALSE, "Boolean 2"=FALSE, "Name"="HHMI - Calibration scan points.vi", "Boolean 3"=FALSE}, {"Boolean"=FALSE, "Boolean 2"=FALSE, "Name"="HHMI - Coerce and Correct Z offset to limits.vi", "Boolean 3"=FALSE}, {"Boolean"=FALSE, "Boolean 2"=FALSE, "Name"="HHMI - Signal vs Z slice functional global.vi", "Boolean 3"=FALSE}, {"Boolean"=FALSE, "Boolean 2"=FALSE, "Name"="HHMI - Current Scan Background ID.vi", "Boolean 3"=FALSE}, {"Boolean"=FALSE, "Boolean 2"=FALSE, "Name"="Load Front Panel control values from cfg file.vi", "Boolean 3"=FALSE}, {"Boolean"=FALSE, "Boolean 2"=FALSE, "Name"="HHMI - Log Image.vi", "Boolean 3"=FALSE}, {"Boolean"=FALSE, "Boolean 2"=FALSE, "Name"="HHMI - Convert Overlap index into subregion indices.vi", "Boolean 3"=FALSE}, {"Boolean"=FALSE, "Boolean 2"=FALSE, "Name"="HHMI - Set XY line pixel size.vi", "Boolean 3"=FALSE}, {"Boolean"=FALSE, "Boolean 2"=FALSE, "Name"="SO Beam expander.lvlib:Pos_Move.vi", "Boolean 3"=FALSE}, {"Boolean"=FALSE, "Boolean 2"=FALSE, "Name"="HHMI - Update X and Y Params from ROI and Pixel Size.vi", "Boolean 3"=FALSE}, {"Boolean"=FALSE, "Boolean 2"=FALSE, "Name"="HHMI - Format phase plot.vi", "Boolean 3"=FALSE}, {"Boolean"=FALSE, "Boolean 2"=FALSE, "Name"="HHMI - Read U16 .tif file and convert to I16 pixels.vi", "Boolean 3"=FALSE}, {"Boolean"=FALSE, "Boolean 2"=FALSE, "Name"="POS?.vi", "Boolean 3"=FALSE}, {"Boolean"=FALSE, "Boolean 2"=FALSE, "Name"="TMX?.vi", "Boolean 3"=FALSE}, {"Boolean"=FALSE, "Boolean 2"=FALSE, "Name"="TMN?.vi", "Boolean 3"=FALSE}, {"Boolean"=FALSE, "Boolean 2"=FALSE, "Name"="HHMI - Find optimized phase for subregions based on neighbors.vi", "Boolean 3"=FALSE}, {"Boolean"=FALSE, "Boolean 2"=FALSE, "Name"="HHMI - Image shift via Image Correlation.vi", "Boolean 3"=FALSE}, {"Boolean"=FALSE, "Boolean 2"=FALSE, "Name"="HHMI - Calc optimized offset of subregion using neighboring subregions.vi", "Boolean 3"=FALSE}, {"Boolean"=FALSE, "Boolean 2"=FALSE, "Name"="HHMI - Stop scan.vi", "Boolean 3"=FALSE}, {"Boolean"=FALSE, "Boolean 2"=FALSE, "Name"="HHMI - Search, add, replace in Laser Power storage global.vi", "Boolean 3"=FALSE}, {"Boolean"=FALSE, "Boolean 2"=FALSE, "Name"="CST?.vi", "Boolean 3"=FALSE}, {"Boolean"=FALSE, "Boolean 2"=FALSE, "Name"="HHMI - PI beam reducer In positions functional globali.vi", "Boolean 3"=FALSE}, {"Boolean"=FALSE, "Boolean 2"=FALSE, "Name"="HHMI - Current SLM settings to Sx and Sy.vi", "Boolean 3"=FALSE}, {"Boolean"=FALSE, "Boolean 2"=FALSE, "Name"="STA?.vi", "Boolean 3"=FALSE}, {"Boolean"=FALSE, "Boolean 2"=FALSE, "Name"="HHMI - Forward Pockel Waveform 1 line Sine.vi", "Boolean 3"=FALSE}, {"Boolean"=FALSE, "Boolean 2"=FALSE, "Name"="HHMI - XY Parameters to Image ROI .vi", "Boolean 3"=FALSE}, {"Boolean"=FALSE, "Boolean 2"=FALSE, "Name"="ONT?.vi", "Boolean 3"=FALSE}, {"Boolean"=FALSE, "Boolean 2"=FALSE, "Name"="TRS?.vi", "Boolean 3"=FALSE}, {"Boolean"=FALSE, "Boolean 2"=FALSE, "Name"="RON?.vi", "Boolean 3"=FALSE}, {"Boolean"=FALSE, "Boolean 2"=FALSE, "Name"="LIM?.vi", "Boolean 3"=FALSE}, {"Boolean"=FALSE, "Boolean 2"=FALSE, "Name"="FRF?.vi", "Boolean 3"=FALSE}, {"Boolean"=FALSE, "Boolean 2"=FALSE, "Name"="SVO?.vi", "Boolean 3"=FALSE}, {"Boolean"=FALSE, "Boolean 2"=FALSE, "Name"="HHMI - Check Waveform parameters for errors or warnings.vi", "Boolean 3"=FALSE}, {"Boolean"=FALSE, "Boolean 2"=FALSE, "Name"="SO Beam expander.lvlib:Wait_Stop.vi", "Boolean 3"=FALSE}, {"Boolean"=FALSE, "Boolean 2"=FALSE, "Name"="Backup.vi", "Boolean 3"=FALSE}, {"Boolean"=FALSE, "Boolean 2"=FALSE, "Name"="Plot 3D Polynomial Fit.vi", "Boolean 3"=FALSE}, {"Boolean"=FALSE, "Boolean 2"=FALSE, "Name"="SO Beam expander.lvlib:Load_Pos_Err.vi", "Boolean 3"=FALSE}, {"Boolean"=FALSE, "Boolean 2"=FALSE, "Name"="Extract subimage from montage.vi", "Boolean 3"=FALSE}, {"Boolean"=FALSE, "Boolean 2"=FALSE, "Name"="HHMI - Find Optimized Phase.vi", "Boolean 3"=FALSE}, {"Boolean"=FALSE, "Boolean 2"=FALSE, "Name"="HHMI - Iterate Mask until um is satisfied.vi", "Boolean 3"=FALSE}, {"Boolean"=FALSE, "Boolean 2"=FALSE, "Name"="RON.vi", "Boolean 3"=FALSE}, {"Boolean"=FALSE, "Boolean 2"=FALSE, "Name"="SVO.vi", "Boolean 3"=FALSE}, {"Boolean"=FALSE, "Boolean 2"=FALSE, "Name"="HHMI - Change clicked subregion by 2pi.vi", "Boolean 3"=FALSE}, {"Boolean"=FALSE, "Boolean 2"=FALSE, "Name"="Define axes to command from boolean array.vi", "Boolean 3"=FALSE}, {"Boolean"=FALSE, "Boolean 2"=FALSE, "Name"="HHMI - Set Safe State.vi", "Boolean 3"=FALSE}, {"Boolean"=FALSE, "Boolean 2"=FALSE, "Name"="HHMI - Correct Linescan Settings.vi", "Boolean 3"=FALSE}, {"Boolean"=FALSE, "Boolean 2"=FALSE, "Name"="HHMI - Border plus 1 pixel arrays.vi", "Boolean 3"=FALSE}, {"Boolean"=FALSE, "Boolean 2"=FALSE, "Name"="HHMI - Laser Calibration to plane coeffs.vi", "Boolean 3"=FALSE}, {"Boolean"=FALSE, "Boolean 2"=FALSE, "Name"="HHMI - Z startup values for XYlineZ GUI.vi", "Boolean 3"=FALSE}, {"Boolean"=FALSE, "Boolean 2"=FALSE, "Name"="HHMI - Load image for Reviewer.vi", "Boolean 3"=FALSE}, {"Boolean"=FALSE, "Boolean 2"=FALSE, "Name"="su10x Configure Smart Shutter.vi", "Boolean 3"=FALSE}, {"Boolean"=FALSE, "Boolean 2"=FALSE, "Name"="HHMI - Generate constant Z array.vi", "Boolean 3"=FALSE}, {"Boolean"=FALSE, "Boolean 2"=FALSE, "Name"="HHMI - PI Read Position.vi", "Boolean 3"=FALSE}, {"Boolean"=FALSE, "Boolean 2"=FALSE, "Name"="HHMI - Generate R Theta coordinate mesh.vi", "Boolean 3"=FALSE}, {"Boolean"=FALSE, "Boolean 2"=FALSE, "Name"="HHMI - Start scan.vi", "Boolean 3"=FALSE}, {"Boolean"=FALSE, "Boolean 2"=FALSE, "Name"="Popup to get 2 Pi value.vi", "Boolean 3"=FALSE}, {"Boolean"=FALSE, "Boolean 2"=FALSE, "Name"="HHMI - Frame averaging functional global.vi", "Boolean 3"=FALSE}, {"Boolean"=FALSE, "Boolean 2"=FALSE, "Name"="HHMI - Pixels to Img Buffer.vi", "Boolean 3"=FALSE}, {"Boolean"=FALSE, "Boolean 2"=FALSE, "Name"="HHMI - Unwrap Phase down the rows of pixels of a single subregion.vi", "Boolean 3"=FALSE}, {"Boolean"=FALSE, "Boolean 2"=FALSE, "Name"="HHMI - Zernike model function and gradient.vi", "Boolean 3"=FALSE}, {"Boolean"=FALSE, "Boolean 2"=FALSE, "Name"="Open or Close front panel of caller.vi", "Boolean 3"=FALSE}, {"Boolean"=FALSE, "Boolean 2"=FALSE, "Name"="HHMI - ExportTable.vi", "Boolean 3"=FALSE}, {"Boolean"=FALSE, "Boolean 2"=FALSE, "Name"="HHMI - Convert SLM mm to stage coords.vi", "Boolean 3"=FALSE}, {"Boolean"=FALSE, "Boolean 2"=FALSE, "Name"="HHMI - Cal Zernike Radial part.vi", "Boolean 3"=FALSE}, {"Boolean"=FALSE, "Boolean 2"=FALSE, "Name"="HHMI - Correct data for position.vi", "Boolean 3"=FALSE}, {"Boolean"=FALSE, "Boolean 2"=FALSE, "Name"="HHMI - Solenoid movement time.vi", "Boolean 3"=FALSE}, {"Boolean"=FALSE, "Boolean 2"=FALSE, "Name"="Commanded axes connected?.vi", "Boolean 3"=FALSE}, {"Boolean"=FALSE, "Boolean 2"=FALSE, "Name"="Generate H Matrix for Least Squares Fit.vi", "Boolean 3"=FALSE}, {"Boolean"=FALSE, "Boolean 2"=FALSE, "Name"="HHMI - Is signal enough.vi", "Boolean 3"=FALSE}, {"Boolean"=FALSE, "Boolean 2"=FALSE, "Name"="HHMI - Set initial SLM image for AO Scan.vi", "Boolean 3"=FALSE}, {"Boolean"=FALSE, "Boolean 2"=FALSE, "Name"="HHMI - Enable disable depending on Acquisition type.vi", "Boolean 3"=FALSE}, {"Boolean"=FALSE, "Boolean 2"=FALSE, "Name"="HHMI - Phase offsets for phase optimization.vi", "Boolean 3"=FALSE}, {"Boolean"=FALSE, "Boolean 2"=FALSE, "Name"="HHMI - Display Bar Graph.vi", "Boolean 3"=FALSE}, {"Boolean"=FALSE, "Boolean 2"=FALSE, "Name"="HHMI - Save Image from Zernike GUI.vi", "Boolean 3"=FALSE}, {"Boolean"=FALSE, "Boolean 2"=FALSE, "Name"="HHMI - Wait for x frames.vi", "Boolean 3"=FALSE}, {"Boolean"=FALSE, "Boolean 2"=FALSE, "Name"="HHMI - Remove Rectangle ROIs.vi", "Boolean 3"=FALSE}, {"Boolean"=FALSE, "Boolean 2"=FALSE, "Name"="HHMI - Copy current background to or from storage cluster.vi", "Boolean 3"=FALSE}, {"Boolean"=FALSE, "Boolean 2"=FALSE, "Name"="HHMI - Enough memory to output full waveform.vi", "Boolean 3"=FALSE}, {"Boolean"=FALSE, "Boolean 2"=FALSE, "Name"="HHMI - Dynamically launch Motion GUI.vi", "Boolean 3"=FALSE}, {"Boolean"=FALSE, "Boolean 2"=FALSE, "Name"="HHMI - Convert Displacement Data to Calibration Array.vi", "Boolean 3"=FALSE}, {"Boolean"=FALSE, "Boolean 2"=FALSE, "Name"="HHMI - Slow axis return create array.vi", "Boolean 3"=FALSE}, {"Boolean"=FALSE, "Boolean 2"=FALSE, "Name"="HHMI - Minimize Chi Square.vi", "Boolean 3"=FALSE}, {"Boolean"=FALSE, "Boolean 2"=FALSE, "Name"="HHMI - Change clicked subregion to NaN.vi", "Boolean 3"=FALSE}, {"Boolean"=FALSE, "Boolean 2"=FALSE, "Name"="Build command substring.vi", "Boolean 3"=FALSE}, {"Boolean"=FALSE, "Boolean 2"=FALSE, "Name"="HHMI - DAQ Initialize all.vi", "Boolean 3"=FALSE}, {"Boolean"=FALSE, "Boolean 2"=FALSE, "Name"="Define connected axes.vi", "Boolean 3"=FALSE}, {"Boolean"=FALSE, "Boolean 2"=FALSE, "Name"="SO Beam expander.lvlib:Control LEDs.vi", "Boolean 3"=FALSE}, {"Boolean"=FALSE, "Boolean 2"=FALSE, "Name"="HHMI - Initialize Image buffers.vi", "Boolean 3"=FALSE}, {"Boolean"=FALSE, "Boolean 2"=FALSE, "Name"="HHMI - Beam reducer control.vi", "Boolean 3"=FALSE}, {"Boolean"=FALSE, "Boolean 2"=FALSE, "Name"="HHMI - Generate Zernike n and m indices.vi", "Boolean 3"=FALSE}, {"Boolean"=FALSE, "Boolean 2"=FALSE, "Name"="HHMI - Set filter wheel and PD for requested PD.vi", "Boolean 3"=FALSE}, {"Boolean"=FALSE, "Boolean 2"=FALSE, "Name"="HHMI - Subregion index storage array.vi", "Boolean 3"=FALSE}, {"Boolean"=FALSE, "Boolean 2"=FALSE, "Name"="HHMI - Crop SLM image to subregions.vi", "Boolean 3"=FALSE}, {"Boolean"=FALSE, "Boolean 2"=FALSE, "Name"="HHMI - AO state functional global.vi", "Boolean 3"=FALSE}, {"Boolean"=FALSE, "Boolean 2"=FALSE, "Name"="Define connected systems (Array).vi", "Boolean 3"=FALSE}, {"Boolean"=FALSE, "Boolean 2"=FALSE, "Name"="HHMI - Set filter to nearest open position.vi", "Boolean 3"=FALSE}, {"Boolean"=FALSE, "Boolean 2"=FALSE, "Name"="HHMI - Analyze Image.vi", "Boolean 3"=FALSE}, {"Boolean"=FALSE, "Boolean 2"=FALSE, "Name"="HHMI - Iterate Mask until N loops.vi", "Boolean 3"=FALSE}, {"Boolean"=FALSE, "Boolean 2"=FALSE, "Name"="HHMI - Reconstruct_Phase_Array_Neal_Algorithm.vi", "Boolean 3"=FALSE}, {"Boolean"=FALSE, "Boolean 2"=FALSE, "Name"="SO Beam expander.lvlib:Init_Motors.vi", "Boolean 3"=FALSE}, {"Boolean"=FALSE, "Boolean 2"=FALSE, "Name"="HHMI - Save image.vi", "Boolean 3"=FALSE}, {"Boolean"=FALSE, "Boolean 2"=FALSE, "Name"="HHMI - Copy Data image buffer to display buffer.vi", "Boolean 3"=FALSE}, {"Boolean"=FALSE, "Boolean 2"=FALSE, "Name"="HHMI - Convert DBL 2D array to U8 2D array and wrap at 2Pi.vi", "Boolean 3"=FALSE}, {"Boolean"=FALSE, "Boolean 2"=FALSE, "Name"="HHMI - Display SLM image.vi", "Boolean 3"=FALSE}, {"Boolean"=FALSE, "Boolean 2"=FALSE, "Name"="Analog Receive String.vi", "Boolean 3"=FALSE}, {"Boolean"=FALSE, "Boolean 2"=FALSE, "Name"="HHMI - Center of Mass Preferences.vi", "Boolean 3"=FALSE}, {"Boolean"=FALSE, "Boolean 2"=FALSE, "Name"="HHMI - Move Laser to mask.vi", "Boolean 3"=FALSE}, {"Boolean"=FALSE, "Boolean 2"=FALSE, "Name"="HHMI - ReadWrite Image Scaling Info.vi", "Boolean 3"=FALSE}, {"Boolean"=FALSE, "Boolean 2"=FALSE, "Name"="HHMI - Analysis Info to String Array.vi", "Boolean 3"=FALSE}, {"Boolean"=FALSE, "Boolean 2"=FALSE, "Name"="Backup to zip.vi", "Boolean 3"=FALSE}, {"Boolean"=FALSE, "Boolean 2"=FALSE, "Name"="HHMI - Calculate phase difference.vi", "Boolean 3"=FALSE}, {"Boolean"=FALSE, "Boolean 2"=FALSE, "Name"="HHMI - Find Brightest pixel.vi", "Boolean 3"=FALSE}, {"Boolean"=FALSE, "Boolean 2"=FALSE, "Name"="HHMI - Maximize window location.vi", "Boolean 3"=FALSE}, {"Boolean"=FALSE, "Boolean 2"=FALSE, "Name"="HHMI - Convert filename base to final filenames.vi", "Boolean 3"=FALSE}, {"Boolean"=FALSE, "Boolean 2"=FALSE, "Name"="HHMI - Calculate inferred image for simplified inverse.vi", "Boolean 3"=FALSE}, {"Boolean"=FALSE, "Boolean 2"=FALSE, "Name"="Zip folder or file.vi", "Boolean 3"=FALSE}, {"Boolean"=FALSE, "Boolean 2"=FALSE, "Name"="32 bit tiff reader.lvlib:Read IFD Entry.vi", "Boolean 3"=FALSE}, {"Boolean"=FALSE, "Boolean 2"=FALSE, "Name"="HHMI - Generate ramp.vi", "Boolean 3"=FALSE}, {"Boolean"=FALSE, "Boolean 2"=FALSE, "Name"="HHMI - Configure SLM for AO Scan.vi", "Boolean 3"=FALSE}, {"Boolean"=FALSE, "Boolean 2"=FALSE, "Name"="HHMI - Center of mass.vi", "Boolean 3"=FALSE}, {"Boolean"=FALSE, "Boolean 2"=FALSE, "Name"="HHMI - Output scan speed control caption.vi", "Boolean 3"=FALSE}, {"Boolean"=FALSE, "Boolean 2"=FALSE, "Name"="HHMI - Running Center of mass subvi.vi", "Boolean 3"=FALSE}, {"Boolean"=FALSE, "Boolean 2"=FALSE, "Name"="HHMI - Border pixel arrays.vi", "Boolean 3"=FALSE}, {"Boolean"=FALSE, "Boolean 2"=FALSE, "Name"="Select values for chosen axes.vi", "Boolean 3"=FALSE}, {"Boolean"=FALSE, "Boolean 2"=FALSE, "Name"="HHMI - Generate length scale.vi", "Boolean 3"=FALSE}, {"Boolean"=FALSE, "Boolean 2"=FALSE, "Name"="HHMI - Correct and Adjust tilt for subregion.vi", "Boolean 3"=FALSE}, {"Boolean"=FALSE, "Boolean 2"=FALSE, "Name"="HHMI - Find bordering subregions using settings.vi", "Boolean 3"=FALSE}, {"Boolean"=FALSE, "Boolean 2"=FALSE, "Name"="Mouse Module.vi", "Boolean 3"=FALSE}, {"Boolean"=FALSE, "Boolean 2"=FALSE, "Name"="FRF.vi", "Boolean 3"=FALSE}, {"Boolean"=FALSE, "Boolean 2"=FALSE, "Name"="FPL.vi", "Boolean 3"=FALSE}, {"Boolean"=FALSE, "Boolean 2"=FALSE, "Name"="FNL.vi", "Boolean 3"=FALSE}, {"Boolean"=FALSE, "Boolean 2"=FALSE, "Name"="HLT.vi", "Boolean 3"=FALSE}, {"Boolean"=FALSE, "Boolean 2"=FALSE, "Name"="GCSTranslateError.vi", "Boolean 3"=FALSE}, {"Boolean"=FALSE, "Boolean 2"=FALSE, "Name"="HHMI - Convert SLM mm to stage coords via linear calc.vi", "Boolean 3"=FALSE}, {"Boolean"=FALSE, "Boolean 2"=FALSE, "Name"="SO Beam expander.lvlib:Serial Read_Timeout.vi", "Boolean 3"=FALSE}, {"Boolean"=FALSE, "Boolean 2"=FALSE, "Name"="HHMI - AO OL Reconstruct wavefront and apply to optimized regions.vi", "Boolean 3"=FALSE}, {"Boolean"=FALSE, "Boolean 2"=FALSE, "Name"="MOV.vi", "Boolean 3"=FALSE}, {"Boolean"=FALSE, "Boolean 2"=FALSE, "Name"="Get arrays without blanks.vi", "Boolean 3"=FALSE}, {"Boolean"=FALSE, "Boolean 2"=FALSE, "Name"="HHMI - Check if centering the scan at the input pixels will be out of range.vi", "Boolean 3"=FALSE}, {"Boolean"=FALSE, "Boolean 2"=FALSE, "Name"="HHMI - Dynamically launch Reviewer.vi", "Boolean 3"=FALSE}, {"Boolean"=FALSE, "Boolean 2"=FALSE, "Name"="HHMI - AO nonOL Reconstruct wavefront and apply to optimized regions.vi", "Boolean 3"=FALSE}, {"Boolean"=FALSE, "Boolean 2"=FALSE, "Name"="HHMI - Make new Filename.vi", "Boolean 3"=FALSE}, {"Boolean"=FALSE, "Boolean 2"=FALSE, "Name"="HHMI - Set COM for extracted montage image.vi", "Boolean 3"=FALSE}, {"Boolean"=FALSE, "Boolean 2"=FALSE, "Name"="HHMI - Dynamically launch SLM Utility.vi", "Boolean 3"=FALSE}, {"Boolean"=FALSE, "Boolean 2"=FALSE, "Name"="HHMI - Dynamically launch Zernike GUI.vi", "Boolean 3"=FALSE}, {"Boolean"=FALSE, "Boolean 2"=FALSE, "Name"="SO Beam expander.lvlib:InterpolateM1M2.vi", "Boolean 3"=FALSE}, {"Boolean"=FALSE, "Boolean 2"=FALSE, "Name"="HHMI - Generate shifted arrays.vi", "Boolean 3"=FALSE}, {"Boolean"=FALSE, "Boolean 2"=FALSE, "Name"="Build query command substring.vi", "Boolean 3"=FALSE}, {"Boolean"=FALSE, "Boolean 2"=FALSE, "Name"="HHMI - Set N subregions.vi", "Boolean 3"=FALSE}, {"Boolean"=FALSE, "Boolean 2"=FALSE, "Name"="HHMI - Calculate Signal from image.vi", "Boolean 3"=FALSE}, {"Boolean"=FALSE, "Boolean 2"=FALSE, "Name"="HHMI - Check AO beam sizes.vi", "Boolean 3"=FALSE}, {"Boolean"=FALSE, "Boolean 2"=FALSE, "Name"="INI Read write dbl.vi", "Boolean 3"=FALSE}, {"Boolean"=FALSE, "Boolean 2"=FALSE, "Name"="HHMI - Convert scaled DBL pixel data to I16.vi", "Boolean 3"=FALSE}, {"Boolean"=FALSE, "Boolean 2"=FALSE, "Name"="HHMI - Slow axis return for ramp.vi", "Boolean 3"=FALSE}, {"Boolean"=FALSE, "Boolean 2"=FALSE, "Name"="HHMI - Generate search parameters to find minimum chi square.vi", "Boolean 3"=FALSE}, {"Boolean"=FALSE, "Boolean 2"=FALSE, "Name"="HHMI - Convert ROI to Point.vi", "Boolean 3"=FALSE}, {"Boolean"=FALSE, "Boolean 2"=FALSE, "Name"="HHMI - Use COM Ref as Signal window center", "Boolean 3"=FALSE}, {"Boolean"=FALSE, "Boolean 2"=FALSE, "Name"="HHMI - Convert Volts to I16 Span.vi", "Boolean 3"=FALSE}, {"Boolean"=FALSE, "Boolean 2"=FALSE, "Name"="HHMI - Optimize offset of mask using neighbors.vi", "Boolean 3"=FALSE}, {"Boolean"=FALSE, "Boolean 2"=FALSE, "Name"="HHMI - Check if SLM ready for Alignment scan.vi", "Boolean 3"=FALSE}, {"Boolean"=FALSE, "Boolean 2"=FALSE, "Name"="HHMI - XY Position lag in pixels.vi", "Boolean 3"=FALSE}, {"Boolean"=FALSE, "Boolean 2"=FALSE, "Name"="HHMI - Set Optimized Phase of current mask as Optimized Beamlets.vi", "Boolean 3"=FALSE}, {"Boolean"=FALSE, "Boolean 2"=FALSE, "Name"="HHMI - Move Laser to subregions.vi", "Boolean 3"=FALSE}, {"Boolean"=FALSE, "Boolean 2"=FALSE, "Name"="Wait for controller ready.vi", "Boolean 3"=FALSE}, {"Boolean"=FALSE, "Boolean 2"=FALSE, "Name"="HHMI - Generate pixel position grid.vi", "Boolean 3"=FALSE}, {"Boolean"=FALSE, "Boolean 2"=FALSE, "Name"="HHMI - Save SLM image to file.vi", "Boolean 3"=FALSE}, {"Boolean"=FALSE, "Boolean 2"=FALSE, "Name"="32 bit tiff reader.lvlib:Read Image File Directory.vi", "Boolean 3"=FALSE}, {"Boolean"=FALSE, "Boolean 2"=FALSE, "Name"="Set Window location.vi", "Boolean 3"=FALSE}, {"Boolean"=FALSE, "Boolean 2"=FALSE, "Name"="HHMI - Forward Pockel Waveform 1 line Ramp.vi", "Boolean 3"=FALSE}, {"Boolean"=FALSE, "Boolean 2"=FALSE, "Name"="HHMI - Merge I16 image and overlay into U64 RGB buffer.vi", "Boolean 3"=FALSE}, {"Boolean"=FALSE, "Boolean 2"=FALSE, "Name"="HHMI - Set mask.vi", "Boolean 3"=FALSE}, {"Boolean"=FALSE, "Boolean 2"=FALSE, "Name"="HHMI - Covert Zmode Coeffs into image.vi", "Boolean 3"=FALSE}, {"Boolean"=FALSE, "Boolean 2"=FALSE, "Name"="HHMI - Fast Axis Cubic Ramp Coeffs.vi", "Boolean 3"=FALSE}, {"Boolean"=FALSE, "Boolean 2"=FALSE, "Name"="HHMI - Initialize all motors.vi", "Boolean 3"=FALSE}, {"Boolean"=FALSE, "Boolean 2"=FALSE, "Name"="HHMI - Current Mask index.vi", "Boolean 3"=FALSE}, {"Boolean"=FALSE, "Boolean 2"=FALSE, "Name"="HHMI - Distance from SLM origin to center of subregion.vi", "Boolean 3"=FALSE}, {"Boolean"=FALSE, "Boolean 2"=FALSE, "Name"="HHMI - Waveform Parameters functional global.vi", "Boolean 3"=FALSE}, {"Boolean"=FALSE, "Boolean 2"=FALSE, "Name"="HHMI - Add Image Correlation Shift to image buffer.vi", "Boolean 3"=FALSE}, {"Boolean"=FALSE, "Boolean 2"=FALSE, "Name"="HHMI - Generate checkerboard.vi", "Boolean 3"=FALSE}, {"Boolean"=FALSE, "Boolean 2"=FALSE, "Name"="HHMI - Duplicate rows in a 2D array (I32).vi", "Boolean 3"=FALSE}, {"Boolean"=FALSE, "Boolean 2"=FALSE, "Name"="HHMI - Table to filenames.vi", "Boolean 3"=FALSE}, {"Boolean"=FALSE, "Boolean 2"=FALSE, "Name"="HHMI - Overlap region definition.vi", "Boolean 3"=FALSE}, {"Boolean"=FALSE, "Boolean 2"=FALSE, "Name"="HHMI - Mask around coords.vi", "Boolean 3"=FALSE}, {"Boolean"=FALSE, "Boolean 2"=FALSE, "Name"="HHMI - Set Valid Number of Samples to write.vi", "Boolean 3"=FALSE}, {"Boolean"=FALSE, "Boolean 2"=FALSE, "Name"="HHMI - Clear other ROIs.vi", "Boolean 3"=FALSE}, {"Boolean"=FALSE, "Boolean 2"=FALSE, "Name"="HHMI - DAQ Close all.vi", "Boolean 3"=FALSE}, {"Boolean"=FALSE, "Boolean 2"=FALSE, "Name"="HHMI - Phase Center coords.vi", "Boolean 3"=FALSE}, {"Boolean"=FALSE, "Boolean 2"=FALSE, "Name"="HHMI - AO move Laser beam on SLM.vi", "Boolean 3"=FALSE}, {"Boolean"=FALSE, "Boolean 2"=FALSE, "Name"="HHMI - Store optimized subregion.vi", "Boolean 3"=FALSE}, {"Boolean"=FALSE, "Boolean 2"=FALSE, "Name"="Analog Functions.vi", "Boolean 3"=FALSE}, {"Boolean"=FALSE, "Boolean 2"=FALSE, "Name"="HHMI - Optimize offset of multiple subregions using neighbors using currently displayed SLM image.vi", "Boolean 3"=FALSE}, {"Boolean"=FALSE, "Boolean 2"=FALSE, "Name"="HHMI - Are there Subregions left.vi", "Boolean 3"=FALSE}, {"Boolean"=FALSE, "Boolean 2"=FALSE, "Name"="SO Beam expander.lvlib:Wait_Home.vi", "Boolean 3"=FALSE}, {"Boolean"=FALSE, "Boolean 2"=FALSE, "Name"="HHMI - Set mask phase.vi", "Boolean 3"=FALSE}, {"Boolean"=FALSE, "Boolean 2"=FALSE, "Name"="HHMI - Beamlet shift calibration functional global.vi", "Boolean 3"=FALSE}, {"Boolean"=FALSE, "Boolean 2"=FALSE, "Name"="SO Beam expander.lvlib:Vel_Move.vi", "Boolean 3"=FALSE}, {"Boolean"=FALSE, "Boolean 2"=FALSE, "Name"="SO Beam expander.lvlib:Motor_Stop.vi", "Boolean 3"=FALSE}, {"Boolean"=FALSE, "Boolean 2"=FALSE, "Name"="HHMI - Convert DBL array to U8 array and wrap at 2Pi.vi", "Boolean 3"=FALSE}, {"Boolean"=FALSE, "Boolean 2"=FALSE, "Name"="HHMI - Copy Full XY Scan buffer to XY Scan buffer.vi", "Boolean 3"=FALSE}, {"Boolean"=FALSE, "Boolean 2"=FALSE, "Name"="HHMI - PI beam reducer Out position functional globali.vi", "Boolean 3"=FALSE}, {"Boolean"=FALSE, "Boolean 2"=FALSE, "Name"="HHMI - Apply Gaussian weight to image.vi", "Boolean 3"=FALSE}, {"Boolean"=FALSE, "Boolean 2"=FALSE, "Name"="HHMI - SLM origin in stage mm.vi", "Boolean 3"=FALSE}, {"Boolean"=FALSE, "Boolean 2"=FALSE, "Name"="HHMI - Store mask set as optimized if improved.vi", "Boolean 3"=FALSE}, {"Boolean"=FALSE, "Boolean 2"=FALSE, "Name"="su10x Configure Filter Wheel.vi", "Boolean 3"=FALSE}, {"Boolean"=FALSE, "Boolean 2"=FALSE, "Name"="HHMI - Check if valid images.vi", "Boolean 3"=FALSE}, {"Boolean"=FALSE, "Boolean 2"=FALSE, "Name"="HHMI - Check if subregion is the center subregion.vi", "Boolean 3"=FALSE}, {"Boolean"=FALSE, "Boolean 2"=FALSE, "Name"="HHMI - Time elasped.vi", "Boolean 3"=FALSE}, {"Boolean"=FALSE, "Boolean 2"=FALSE, "Name"="HHMI - Pause GUI and update waveform.vi", "Boolean 3"=FALSE}, {"Boolean"=FALSE, "Boolean 2"=FALSE, "Name"="HHMI - Create Gaussian weighting functions.vi", "Boolean 3"=FALSE}, {"Boolean"=FALSE, "Boolean 2"=FALSE, "Name"="HHMI - Duplicate single line data.vi", "Boolean 3"=FALSE}, {"Boolean"=FALSE, "Boolean 2"=FALSE, "Name"="HHMI - I16 PNG to U16 TIF converter.vi", "Boolean 3"=FALSE}, {"Boolean"=FALSE, "Boolean 2"=FALSE, "Name"="HHMI - Enable disable depending on AO algo.vi", "Boolean 3"=FALSE}, {"Boolean"=FALSE, "Boolean 2"=FALSE, "Name"="HHMI - Iterate and obtain Phi.vi", "Boolean 3"=FALSE}, {"Boolean"=FALSE, "Boolean 2"=FALSE, "Name"="HHMI - Calculate error between 1st half and 2nd half of SLM on.vi", "Boolean 3"=FALSE}, {"Boolean"=FALSE, "Boolean 2"=FALSE, "Name"="HHMI - Joystick button definitions.vi", "Boolean 3"=FALSE}, {"Boolean"=FALSE, "Boolean 2"=FALSE, "Name"="#7.vi", "Boolean 3"=FALSE}, {"Boolean"=FALSE, "Boolean 2"=FALSE, "Name"="HHMI - Set SLM for montage.vi", "Boolean 3"=FALSE}, {"Boolean"=FALSE, "Boolean 2"=FALSE, "Name"="HHMI - Smooth Image.vi", "Boolean 3"=FALSE}, {"Boolean"=FALSE, "Boolean 2"=FALSE, "Name"="Find project reference.vi", "Boolean 3"=FALSE}, {"Boolean"=FALSE, "Boolean 2"=FALSE, "Name"="HHMI - Calculate bjk.vi", "Boolean 3"=FALSE}, {"Boolean"=FALSE, "Boolean 2"=FALSE, "Name"="ERR?.vi", "Boolean 3"=FALSE}, {"Boolean"=FALSE, "Boolean 2"=FALSE, "Name"="SO Beam expander.lvlib:Read M1M2 Position.vi", "Boolean 3"=FALSE}, {"Boolean"=FALSE, "Boolean 2"=FALSE, "Name"="HHMI - Create N Buffer images - keep reference.vi", "Boolean 3"=FALSE}, {"Boolean"=FALSE, "Boolean 2"=FALSE, "Name"="HHMI - Read Pixel sizes from image.vi", "Boolean 3"=FALSE}, {"Boolean"=FALSE, "Boolean 2"=FALSE, "Name"="HHMI - Generate random pattern.vi", "Boolean 3"=FALSE}, {"Boolean"=FALSE, "Boolean 2"=FALSE, "Name"="HHMI - Set filename GUI.vi", "Boolean 3"=FALSE}, {"Boolean"=FALSE, "Boolean 2"=FALSE, "Name"="HHMI - Convert DBL to U8 and wrap at 2Pi.vi", "Boolean 3"=FALSE}, {"Boolean"=FALSE, "Boolean 2"=FALSE, "Name"="HHMI - Convert Pixels to XY Parameters.vi", "Boolean 3"=FALSE}, {"Boolean"=FALSE, "Boolean 2"=FALSE, "Name"="HHMI - Optimize offset of subregion using neighbors using currently displayed SLM image.vi", "Boolean 3"=FALSE}, {"Boolean"=FALSE, "Boolean 2"=FALSE, "Name"="HHMI - SLM settings for all on mask phase offset optimization.vi", "Boolean 3"=FALSE}, {"Boolean"=FALSE, "Boolean 2"=FALSE, "Name"="Open Folder in Explorer Window.vi", "Boolean 3"=FALSE}, {"Boolean"=FALSE, "Boolean 2"=FALSE, "Name"="HHMI - Correct Z Stack Settings.vi", "Boolean 3"=FALSE}, {"Boolean"=FALSE, "Boolean 2"=FALSE, "Name"="HHMI - Reset Scan Modules.vi", "Boolean 3"=FALSE}, {"Boolean"=FALSE, "Boolean 2"=FALSE, "Name"="HHMI - Are there Masks left.vi", "Boolean 3"=FALSE}, {"Boolean"=FALSE, "Boolean 2"=FALSE, "Name"="HHMI - Convert arrays to subregion array.vi", "Boolean 3"=FALSE}, {"Boolean"=FALSE, "Boolean 2"=FALSE, "Name"="HHMI - Update all subregions.vi", "Boolean 3"=FALSE}, {"Boolean"=FALSE, "Boolean 2"=FALSE, "Name"="HHMI - Export SLM image.vi", "Boolean 3"=FALSE}, {"Boolean"=FALSE, "Boolean 2"=FALSE, "Name"="HHMI - Store multiple subregions as optimized.vi", "Boolean 3"=FALSE}, {"Boolean"=FALSE, "Boolean 2"=FALSE, "Name"="HHMI - Generate binary.vi", "Boolean 3"=FALSE}, {"Boolean"=FALSE, "Boolean 2"=FALSE, "Name"="HHMI - Generate starting pattern for phase match algorithm.vi", "Boolean 3"=FALSE}, {"Boolean"=FALSE, "Boolean 2"=FALSE, "Name"="HHMI - Subtract background image from data.vi", "Boolean 3"=FALSE}, {"Boolean"=FALSE, "Boolean 2"=FALSE, "Name"="HHMI - Integrator Timebase.vi", "Boolean 3"=FALSE}, {"Boolean"=FALSE, "Boolean 2"=FALSE, "Name"="HHMI - Is Joystick action needed.vi", "Boolean 3"=FALSE}, {"Boolean"=FALSE, "Boolean 2"=FALSE, "Name"="HHMI - Target signal during AO scan.vi", "Boolean 3"=FALSE}, {"Boolean"=FALSE, "Boolean 2"=FALSE, "Name"="#5_old.vi", "Boolean 3"=FALSE}, {"Boolean"=FALSE, "Boolean 2"=FALSE, "Name"="#5.vi", "Boolean 3"=FALSE}, {"Boolean"=FALSE, "Boolean 2"=FALSE, "Name"="SO Beam expander.lvlib:Wait+ (ms).vi", "Boolean 3"=FALSE}, {"Boolean"=FALSE, "Boolean 2"=FALSE, "Name"="HHMI - Linescan settings functional global.vi", "Boolean 3"=FALSE}, {"Boolean"=FALSE, "Boolean 2"=FALSE, "Name"="SO Beam expander.lvlib:Set_Home.vi", "Boolean 3"=FALSE}, {"Boolean"=FALSE, "Boolean 2"=FALSE, "Name"="SO Beam expander.lvlib:GenerateM1M2.vi", "Boolean 3"=FALSE}, {"Boolean"=FALSE, "Boolean 2"=FALSE, "Name"="HHMI - Convert to TIF and export to Image J.vi", "Boolean 3"=FALSE}, {"Boolean"=FALSE, "Boolean 2"=FALSE, "Name"="HHMI - Copy Image Display buffer from engine to UI Image Display buffer.vi", "Boolean 3"=FALSE}, {"Boolean"=FALSE, "Boolean 2"=FALSE, "Name"="HHMI - What subregion indices are on.vi", "Boolean 3"=FALSE}, {"Boolean"=FALSE, "Boolean 2"=FALSE, "Name"="HHMI - Undo current mask optimization.vi", "Boolean 3"=FALSE}, {"Boolean"=FALSE, "Boolean 2"=FALSE, "Name"="HHMI - Remove masked points from 1D array.vi", "Boolean 3"=FALSE}, {"Boolean"=FALSE, "Boolean 2"=FALSE, "Name"="HHMI - ReadWrite Image Settings Info.vi", "Boolean 3"=FALSE}, {"Boolean"=FALSE, "Boolean 2"=FALSE, "Name"="HHMI - ReadWrite Channel Info.vi", "Boolean 3"=FALSE}, {"Boolean"=FALSE, "Boolean 2"=FALSE, "Name"="HHMI - SubSubregion index storage array.vi", "Boolean 3"=FALSE}, {"Boolean"=FALSE, "Boolean 2"=FALSE, "Name"="HHMI - Generate initial phase reference pattern.vi", "Boolean 3"=FALSE}, {"Boolean"=FALSE, "Boolean 2"=FALSE, "Name"="Pop-up wait prompt.vi", "Boolean 3"=FALSE}, {"Boolean"=FALSE, "Boolean 2"=FALSE, "Name"="HHMI - Image save is scaled.vi", "Boolean 3"=FALSE}, {"Boolean"=FALSE, "Boolean 2"=FALSE, "Name"="SO Beam expander.lvlib:Home Both.vi", "Boolean 3"=FALSE}, {"Boolean"=FALSE, "Boolean 2"=FALSE, "Name"="HHMI - Set SLM for optimized angle.vi", "Boolean 3"=FALSE}, {"Boolean"=FALSE, "Boolean 2"=FALSE, "Name"="HHMI - Display ROI and tools.vi", "Boolean 3"=FALSE}, {"Boolean"=FALSE, "Boolean 2"=FALSE, "Name"="HHMI - Show scale bar overlay on image.vi", "Boolean 3"=FALSE}, {"Boolean"=FALSE, "Boolean 2"=FALSE, "Name"="HHMI - Set subregion phase.vi", "Boolean 3"=FALSE}, {"Boolean"=FALSE, "Boolean 2"=FALSE, "Name"="Quartz SLM utility.vi:Instance:2", "Boolean 3"=FALSE}, {"Boolean"=FALSE, "Boolean 2"=FALSE, "Name"="Quartz SLM utility.vi:Instance:1", "Boolean 3"=FALSE}, {"Boolean"=FALSE, "Boolean 2"=FALSE, "Name"="Quartz SLM utility.vi:Instance:0", "Boolean 3"=FALSE}, {"Boolean"=FALSE, "Boolean 2"=FALSE, "Name"="Quartz Reviewer.vi:Instance:1", "Boolean 3"=FALSE}, {"Boolean"=FALSE, "Boolean 2"=FALSE, "Name"="TIF conversion GUI.vi:Instance:0", "Boolean 3"=FALSE}, {"Boolean"=FALSE, "Boolean 2"=FALSE, "Name"="HHMI - Analysis Table module.vi:Instance:0", "Boolean 3"=FALSE}, {"Boolean"=FALSE, "Boolean 2"=FALSE, "Name"="HHMI - Make new Filename.vi:Instance:0", "Boolean 3"=FALSE}, {"Boolean"=FALSE, "Boolean 2"=FALSE, "Name"="HHMI - Zernike GUI.vi:Instance:3", "Boolean 3"=FALSE}, {"Boolean"=FALSE, "Boolean 2"=FALSE, "Name"="HHMI - Zernike GUI.vi:Instance:2", "Boolean 3"=FALSE}, {"Boolean"=FALSE, "Boolean 2"=FALSE, "Name"="HHMI - Zernike GUI.vi:Instance:1", "Boolean 3"=FALSE}, {"Boolean"=FALSE, "Boolean 2"=FALSE, "Name"="HHMI - Zernike GUI.vi:Instance:0", "Boolean 3"=FALSE}, {"Boolean"=FALSE, "Boolean 2"=FALSE, "Name"="Save Front Panel controls to cfg file.vi", "Boolean 3"=FALSE}, {"Boolean"=FALSE, "Boolean 2"=FALSE, "Name"="HHMI - Generate row of data for table.vi", "Boolean 3"=FALSE}, {"Boolean"=FALSE, "Boolean 2"=FALSE, "Name"="HHMI - Cal Zernike R theta coords and masked pixels.vi", "Boolean 3"=FALSE}, {"Boolean"=FALSE, "Boolean 2"=FALSE, "Name"="Set GUI origin and window location.vi", "Boolean 3"=FALSE}, {"Boolean"=FALSE, "Boolean 2"=FALSE, "Name"="HHMI - Current Overlap region index.vi", "Boolean 3"=FALSE}, {"Boolean"=FALSE, "Boolean 2"=FALSE, "Name"="HHMI - Correct and set Z Parameters for XYlineZ.vi", "Boolean 3"=FALSE}, {"Boolean"=FALSE, "Boolean 2"=FALSE, "Name"="HHMI - ReadWrite SLMaddedFile Info.vi", "Boolean 3"=FALSE}, {"Boolean"=FALSE, "Boolean 2"=FALSE, "Name"="HHMI - Shutter control.vi", "Boolean 3"=FALSE}, {"Boolean"=FALSE, "Boolean 2"=FALSE, "Name"="HHMI - Fast Axis Waveform 1 line Sine.vi", "Boolean 3"=FALSE}, {"Boolean"=FALSE, "Boolean 2"=FALSE, "Name"="HHMI - Display Images.vi", "Boolean 3"=FALSE}, {"Boolean"=FALSE, "Boolean 2"=FALSE, "Name"="Open files with exe.vi", "Boolean 3"=FALSE}, {"Boolean"=FALSE, "Boolean 2"=FALSE, "Name"="HHMI - Find all valid Digital lines.vi", "Boolean 3"=FALSE}, {"Boolean"=FALSE, "Boolean 2"=FALSE, "Name"="HHMI - Switch pixels to remove fill factor effects.vi", "Boolean 3"=FALSE}, {"Boolean"=FALSE, "Boolean 2"=FALSE, "Name"="HHMI - Check beam sizes if montage.vi", "Boolean 3"=FALSE}, {"Boolean"=FALSE, "Boolean 2"=FALSE, "Name"="SO Beam expander.lvlib:Tweak_Expansion.vi", "Boolean 3"=FALSE}, {"Boolean"=FALSE, "Boolean 2"=FALSE, "Name"="HHMI - Obtain 2 pi value from image or from user popup.vi", "Boolean 3"=FALSE}, {"Boolean"=FALSE, "Boolean 2"=FALSE, "Name"="HHMI - Signal Center Coords functional global.vi", "Boolean 3"=FALSE}, {"Boolean"=FALSE, "Boolean 2"=FALSE, "Name"="HHMI - Generate File paths.vi", "Boolean 3"=FALSE}, {"Boolean"=FALSE, "Boolean 2"=FALSE, "Name"="HHMI - Version info.vi", "Boolean 3"=FALSE}, {"Boolean"=FALSE, "Boolean 2"=FALSE, "Name"="HHMI - Axis limits.vi", "Boolean 3"=FALSE}, {"Boolean"=FALSE, "Boolean 2"=FALSE, "Name"="HHMI - Magnify Image.vi", "Boolean 3"=FALSE}, {"Boolean"=FALSE, "Boolean 2"=FALSE, "Name"="HHMI - Add offset to subregion.vi", "Boolean 3"=FALSE}, {"Boolean"=FALSE, "Boolean 2"=FALSE, "Name"="HHMI - Calculate qjk.vi", "Boolean 3"=FALSE}, {"Boolean"=FALSE, "Boolean 2"=FALSE, "Name"="HHMI - Custom error codes.vi", "Boolean 3"=FALSE}, {"Boolean"=FALSE, "Boolean 2"=FALSE, "Name"="Wait for vi to be running.vi", "Boolean 3"=FALSE}, {"Boolean"=FALSE, "Boolean 2"=FALSE, "Name"="HHMI - I16 Image to U16 TIF file.vi", "Boolean 3"=FALSE}, {"Boolean"=FALSE, "Boolean 2"=FALSE, "Name"="Analog FGlobal.vi", "Boolean 3"=FALSE}, {"Boolean"=FALSE, "Boolean 2"=FALSE, "Name"="HHMI - Turn on center overlap region.vi", "Boolean 3"=FALSE}, {"Boolean"=FALSE, "Boolean 2"=FALSE, "Name"="HHMI - Convert U16 .tif file pixels to I16 pixels if necessary.vi", "Boolean 3"=FALSE}, {"Boolean"=FALSE, "Boolean 2"=FALSE, "Name"="HHMI - Scan Preferences functional global.vi", "Boolean 3"=FALSE}, {"Boolean"=FALSE, "Boolean 2"=FALSE, "Name"="HHMI - Set 1 SLM region.vi", "Boolean 3"=FALSE}, {"Boolean"=FALSE, "Boolean 2"=FALSE, "Name"="HHMI - Are Pixels saturated.vi", "Boolean 3"=FALSE}, {"Boolean"=FALSE, "Boolean 2"=FALSE, "Name"="SO Beam expander.lvlib:Set Mag.vi", "Boolean 3"=FALSE}, {"Boolean"=FALSE, "Boolean 2"=FALSE, "Name"="HHMI - Remove duplicated file paths.vi", "Boolean 3"=FALSE}, {"Boolean"=FALSE, "Boolean 2"=FALSE, "Name"="SO Beam expander.lvlib:Focus_Expansion.vi", "Boolean 3"=FALSE}, {"Boolean"=FALSE, "Boolean 2"=FALSE, "Name"="HHMI - Coerce XY Parameters to limits.vi", "Boolean 3"=FALSE}, {"Boolean"=FALSE, "Boolean 2"=FALSE, "Name"="HHMI - Scale Background to match.vi", "Boolean 3"=FALSE}, {"Boolean"=FALSE, "Boolean 2"=FALSE, "Name"="Assign NaN for chosen axes.vi", "Boolean 3"=FALSE}, {"Boolean"=FALSE, "Boolean 2"=FALSE, "Name"="HHMI - Turn off all subregions.vi", "Boolean 3"=FALSE}, {"Boolean"=FALSE, "Boolean 2"=FALSE, "Name"="SO Beam expander.lvlib:Adjust Mag.vi", "Boolean 3"=FALSE}, {"Boolean"=FALSE, "Boolean 2"=FALSE, "Name"="HHMI - Copy Image pixels into SGL buffer with custom data.vi", "Boolean 3"=FALSE}, {"Boolean"=FALSE, "Boolean 2"=FALSE, "Name"="Pop state off string queue.vi", "Boolean 3"=FALSE}, {"Boolean"=FALSE, "Boolean 2"=FALSE, "Name"="HHMI - PI beam reducer move in or out.vi", "Boolean 3"=FALSE}, {"Boolean"=FALSE, "Boolean 2"=FALSE, "Name"="HHMI - Manually change clicked subregion by 2pi.vi", "Boolean 3"=FALSE}, {"Boolean"=FALSE, "Boolean 2"=FALSE, "Name"="HHMI - Is current mask signal better than what we had previously.vi", "Boolean 3"=FALSE}, {"Boolean"=FALSE, "Boolean 2"=FALSE, "Name"="HHMI - Remove duplicated states.vi", "Boolean 3"=FALSE}, {"Boolean"=FALSE, "Boolean 2"=FALSE, "Name"="HHMI - Copy Data to Full XY Scan buffer if necessary.vi", "Boolean 3"=FALSE}, {"Boolean"=FALSE, "Boolean 2"=FALSE, "Name"="HHMI - Save current SLM display as Optimized.vi", "Boolean 3"=FALSE}, {"Boolean"=FALSE, "Boolean 2"=FALSE, "Name"="HHMI - Overlap wavefront reconstruction settings.vi", "Boolean 3"=FALSE}, {"Boolean"=FALSE, "Boolean 2"=FALSE, "Name"="SO Beam expander.lvlib:Chk_Index.vi", "Boolean 3"=FALSE}, {"Boolean"=FALSE, "Boolean 2"=FALSE, "Name"="HHMI - Center Coordinates to center of image if in Image Correlation.vi", "Boolean 3"=FALSE}, {"Boolean"=FALSE, "Boolean 2"=FALSE, "Name"="HHMI - Subsubregion indices that make up a subregion.vi", "Boolean 3"=FALSE}, {"Boolean"=FALSE, "Boolean 2"=FALSE, "Name"="HHMI - Calculate current normalized signal.vi", "Boolean 3"=FALSE}, {"Boolean"=FALSE, "Boolean 2"=FALSE, "Name"="Pop state off string queue - no rtm.vi", "Boolean 3"=FALSE}, {"Boolean"=FALSE, "Boolean 2"=FALSE, "Name"="OR Error clusters.vi", "Boolean 3"=FALSE}, {"Boolean"=FALSE, "Boolean 2"=FALSE, "Name"="Initialize Global DaisyChain.vi", "Boolean 3"=FALSE}, {"Boolean"=FALSE, "Boolean 2"=FALSE, "Name"="Initialize Global2.vi", "Boolean 3"=FALSE}, {"Boolean"=FALSE, "Boolean 2"=FALSE, "Name"="HHMI - Manually change clicked subregion to NaN.vi", "Boolean 3"=FALSE}, {"Boolean"=FALSE, "Boolean 2"=FALSE, "Name"="HHMI - Convert XY Parameters to ROI Pixels.vi", "Boolean 3"=FALSE}, {"Boolean"=FALSE, "Boolean 2"=FALSE, "Name"="HHMI - Beam sizes during AO scan.vi", "Boolean 3"=FALSE}, {"Boolean"=FALSE, "Boolean 2"=FALSE, "Name"="HHMI - Set SLM for mask phase offset optimization.vi", "Boolean 3"=FALSE}, {"Boolean"=FALSE, "Boolean 2"=FALSE, "Name"="Read all custom data.vi", "Boolean 3"=FALSE}, {"Boolean"=FALSE, "Boolean 2"=FALSE, "Name"="HHMI - Correct power for BR.vi", "Boolean 3"=FALSE}, {"Boolean"=FALSE, "Boolean 2"=FALSE, "Name"="HHMI - Autoscroll.vi", "Boolean 3"=FALSE}, {"Boolean"=FALSE, "Boolean 2"=FALSE, "Name"="32 bit tiff reader.lvlib:Generate Colour Table.vi", "Boolean 3"=FALSE}, {"Boolean"=FALSE, "Boolean 2"=FALSE, "Name"="SO Beam expander.lvlib:Err_Clear.vi", "Boolean 3"=FALSE}, {"Boolean"=FALSE, "Boolean 2"=FALSE, "Name"="HHMI - Angle iteration storage global.vi", "Boolean 3"=FALSE}, {"Boolean"=FALSE, "Boolean 2"=FALSE, "Name"="HHMI - Estimate Phase Fit params.vi", "Boolean 3"=FALSE}, {"Boolean"=FALSE, "Boolean 2"=FALSE, "Name"="Search variant array.vi", "Boolean 3"=FALSE}, {"Boolean"=FALSE, "Boolean 2"=FALSE, "Name"="HHMI - Global ramp current display.vi", "Boolean 3"=FALSE}, {"Boolean"=FALSE, "Boolean 2"=FALSE, "Name"="HHMI - Calculate which borders to ignore.vi", "Boolean 3"=FALSE}, {"Boolean"=FALSE, "Boolean 2"=FALSE, "Name"="Substract axes array subset from axes array.vi", "Boolean 3"=FALSE}, {"Boolean"=FALSE, "Boolean 2"=FALSE, "Name"="Evaluate 3D Polynomial.vi", "Boolean 3"=FALSE}, {"Boolean"=FALSE, "Boolean 2"=FALSE, "Name"="HHMI - Scan type functional global.vi", "Boolean 3"=FALSE}, {"Boolean"=FALSE, "Boolean 2"=FALSE, "Name"="HHMI - Analysis channel buffer and functional global.vi", "Boolean 3"=FALSE}, {"Boolean"=FALSE, "Boolean 2"=FALSE, "Name"="HHMI - Determine COM confidence.vi", "Boolean 3"=FALSE}, {"Boolean"=FALSE, "Boolean 2"=FALSE, "Name"="HHMI - Reject new settings if no improvement during AO scan.vi", "Boolean 3"=FALSE}, {"Boolean"=FALSE, "Boolean 2"=FALSE, "Name"="Circle Mask.vi", "Boolean 3"=FALSE}, {"Boolean"=FALSE, "Boolean 2"=FALSE, "Name"="su10x Configure Shutter.vi", "Boolean 3"=FALSE}, {"Boolean"=FALSE, "Boolean 2"=FALSE, "Name"="SO Beam expander.lvlib:Set_COI.vi", "Boolean 3"=FALSE}, {"Boolean"=FALSE, "Boolean 2"=FALSE, "Name"="SO Beam expander.lvlib:Clear_Home.vi", "Boolean 3"=FALSE}, {"Boolean"=FALSE, "Boolean 2"=FALSE, "Name"="SO Beam expander.lvlib:Clear_COI.vi", "Boolean 3"=FALSE}, {"Boolean"=FALSE, "Boolean 2"=FALSE, "Name"="Wait (ms) with error IO.vi", "Boolean 3"=FALSE}, {"Boolean"=FALSE, "Boolean 2"=FALSE, "Name"="HHMI - Smallest DAQ V and um steps.vi", "Boolean 3"=FALSE}, {"Boolean"=FALSE, "Boolean 2"=FALSE, "Name"="HHMI - AO optimization algorithm functional global.vi", "Boolean 3"=FALSE}, {"Boolean"=FALSE, "Boolean 2"=FALSE, "Name"="HHMI - Duplicate y array data.vi", "Boolean 3"=FALSE}, {"Boolean"=FALSE, "Boolean 2"=FALSE, "Name"="HHMI - Replace extrapolated points with zero.vi", "Boolean 3"=FALSE}, {"Boolean"=FALSE, "Boolean 2"=FALSE, "Name"="HHMI - Copy Img no move overlays.vi", "Boolean 3"=FALSE}, {"Boolean"=FALSE, "Boolean 2"=FALSE, "Name"="HHMI - Coerce but keep overload pixel.vi", "Boolean 3"=FALSE}, {"Boolean"=FALSE, "Boolean 2"=FALSE, "Name"="HHMI - Beam reducer request from Motion GUI functional global.vi", "Boolean 3"=FALSE}, {"Boolean"=FALSE, "Boolean 2"=FALSE, "Name"="32 bit tiff reader.lvlib:PageDialog.vi", "Boolean 3"=FALSE}, {"Boolean"=FALSE, "Boolean 2"=FALSE, "Name"="HHMI - Save current SLM display as Stage 1 optimized.vi", "Boolean 3"=FALSE}, {"Boolean"=FALSE, "Boolean 2"=FALSE, "Name"="HHMI - Power increase or decrease factor.vi", "Boolean 3"=FALSE}, {"Boolean"=FALSE, "Boolean 2"=FALSE, "Name"="HHMI - Scan initialized functional global.vi", "Boolean 3"=FALSE}, {"Boolean"=FALSE, "Boolean 2"=FALSE, "Name"="HHMI - Move laser during AO scan.vi", "Boolean 3"=FALSE}, {"Boolean"=FALSE, "Boolean 2"=FALSE, "Name"="HHMI - Number of subregions on.vi", "Boolean 3"=FALSE}, {"Boolean"=FALSE, "Boolean 2"=FALSE, "Name"="HHMI - Error announcer full message.vi", "Boolean 3"=FALSE}, {"Boolean"=FALSE, "Boolean 2"=FALSE, "Name"="HHMI - Create N image buffers.vi", "Boolean 3"=FALSE}, {"Boolean"=FALSE, "Boolean 2"=FALSE, "Name"="HHMI - Phase Signal Center selection auto or manual.vi", "Boolean 3"=FALSE}, {"Boolean"=FALSE, "Boolean 2"=FALSE, "Name"="HHMI - Beam size enum to DBL converter.vi", "Boolean 3"=FALSE}, {"Boolean"=FALSE, "Boolean 2"=FALSE, "Name"="Write all custom data.vi", "Boolean 3"=FALSE}, {"Boolean"=FALSE, "Boolean 2"=FALSE, "Name"="HHMI - Laser alignment parameters functional global.vi", "Boolean 3"=FALSE}, {"Boolean"=FALSE, "Boolean 2"=FALSE, "Name"="HHMI - Move Laser to SLM center.vi", "Boolean 3"=FALSE}, {"Boolean"=FALSE, "Boolean 2"=FALSE, "Name"="HHMI - Generate Support files File paths.vi", "Boolean 3"=FALSE}, {"Boolean"=FALSE, "Boolean 2"=FALSE, "Name"="SO Beam expander.lvlib:Motor_Off.vi", "Boolean 3"=FALSE}, {"Boolean"=FALSE, "Boolean 2"=FALSE, "Name"="SO Beam expander.lvlib:Motor_On.vi", "Boolean 3"=FALSE}, {"Boolean"=FALSE, "Boolean 2"=FALSE, "Name"="32 bit tiff reader.lvlib:Read Header.vi", "Boolean 3"=FALSE}, {"Boolean"=FALSE, "Boolean 2"=FALSE, "Name"="HHMI - Digital channel lookup.vi", "Boolean 3"=FALSE}, {"Boolean"=FALSE, "Boolean 2"=FALSE, "Name"="HHMI - Overwrite output write buffer.vi", "Boolean 3"=FALSE}, {"Boolean"=FALSE, "Boolean 2"=FALSE, "Name"="SO Beam expander.lvlib:Focus.vi", "Boolean 3"=FALSE}, {"Boolean"=FALSE, "Boolean 2"=FALSE, "Name"="TIF conversion GUI.vi", "Boolean 3"=FALSE}, {"Boolean"=FALSE, "Boolean 2"=FALSE, "Name"="HHMI - Is this mask to be stored.vi", "Boolean 3"=FALSE}, {"Boolean"=FALSE, "Boolean 2"=FALSE, "Name"="HHMI - AO background action.vi", "Boolean 3"=FALSE}, {"Boolean"=FALSE, "Boolean 2"=FALSE, "Name"="HHMI - Add counts to waveforms at beginning and end.vi", "Boolean 3"=FALSE}, {"Boolean"=FALSE, "Boolean 2"=FALSE, "Name"="HHMI - Read last filenames and process into string for table.vi", "Boolean 3"=FALSE}, {"Boolean"=FALSE, "Boolean 2"=FALSE, "Name"="HHMI - Pause after Scan functional global.vi", "Boolean 3"=FALSE}, {"Boolean"=FALSE, "Boolean 2"=FALSE, "Name"="Set Version in titlebar.vi", "Boolean 3"=FALSE}, {"Boolean"=FALSE, "Boolean 2"=FALSE, "Name"="HHMI - Store last scan as reference if in Phase Only mode.vi", "Boolean 3"=FALSE}, {"Boolean"=FALSE, "Boolean 2"=FALSE, "Name"="Copy all custom data.vi", "Boolean 3"=FALSE}, {"Boolean"=FALSE, "Boolean 2"=FALSE, "Name"="HHMI - Generate Y return or flyback for Ramp waveform.vi", "Boolean 3"=FALSE}, {"Boolean"=FALSE, "Boolean 2"=FALSE, "Name"="HHMI - Turn on just Reference Mask of first row.vi", "Boolean 3"=FALSE}, {"Boolean"=FALSE, "Boolean 2"=FALSE, "Name"="HHMI - Version Constant.vi", "Boolean 3"=FALSE}, {"Boolean"=FALSE, "Boolean 2"=FALSE, "Name"="HHMI - Galil has Error", "Boolean 3"=FALSE}, {"Boolean"=FALSE, "Boolean 2"=FALSE, "Name"="Sim and Debug.vi", "Boolean 3"=FALSE}, {"Boolean"=FALSE, "Boolean 2"=FALSE, "Name"="HHMI - Flatten channel ranges to array of strings.vi", "Boolean 3"=FALSE}, {"Boolean"=FALSE, "Boolean 2"=FALSE, "Name"="Clear custom data.vi", "Boolean 3"=FALSE}, {"Boolean"=FALSE, "Boolean 2"=FALSE, "Name"="Find largest peak.vi", "Boolean 3"=FALSE}, {"Boolean"=FALSE, "Boolean 2"=FALSE, "Name"="Decimate 2D array.vi", "Boolean 3"=FALSE}, {"Boolean"=FALSE, "Boolean 2"=FALSE, "Name"="Galil COMMAND.VI", "Boolean 3"=FALSE}, {"Boolean"=FALSE, "Boolean 2"=FALSE, "Name"="HHMI - Image Correlation reference scan reference type.vi", "Boolean 3"=FALSE}, {"Boolean"=FALSE, "Boolean 2"=FALSE, "Name"="HHMI - Center of Display image in pixel indices.vi", "Boolean 3"=FALSE}, {"Boolean"=FALSE, "Boolean 2"=FALSE, "Name"="HHMI - Analysis Constants functional global.vi", "Boolean 3"=FALSE}, {"Boolean"=FALSE, "Boolean 2"=FALSE, "Name"="Reshape 2D array to 1D subregion.vi", "Boolean 3"=FALSE}, {"Boolean"=FALSE, "Boolean 2"=FALSE, "Name"="Create folder if it doesn't exist.vi", "Boolean 3"=FALSE}, {"Boolean"=FALSE, "Boolean 2"=FALSE, "Name"="HHMI - Coerce slow axis XYZ params.vi", "Boolean 3"=FALSE}, {"Boolean"=FALSE, "Boolean 2"=FALSE, "Name"="*IDN?.vi", "Boolean 3"=FALSE}, {"Boolean"=FALSE, "Boolean 2"=FALSE, "Name"="Galil OPEN.VI", "Boolean 3"=FALSE}, {"Boolean"=FALSE, "Boolean 2"=FALSE, "Name"="HHMI - Find Max laser power wrapper.vi", "Boolean 3"=FALSE}, {"Boolean"=FALSE, "Boolean 2"=FALSE, "Name"="Clear Image buffer.vi", "Boolean 3"=FALSE}, {"Boolean"=FALSE, "Boolean 2"=FALSE, "Name"="HHMI - Pre-Mask signal storage global.vi", "Boolean 3"=FALSE}, {"Boolean"=FALSE, "Boolean 2"=FALSE, "Name"="su10x Control Mode.vi", "Boolean 3"=FALSE}, {"Boolean"=FALSE, "Boolean 2"=FALSE, "Name"="HHMI - Use FFT image recovery.vi", "Boolean 3"=FALSE}, {"Boolean"=FALSE, "Boolean 2"=FALSE, "Name"="HHMI - Any Border pixel array NaN.vi", "Boolean 3"=FALSE}, {"Boolean"=FALSE, "Boolean 2"=FALSE, "Name"="Convert radians to degrees.vi", "Boolean 3"=FALSE}, {"Boolean"=FALSE, "Boolean 2"=FALSE, "Name"="HHMI - User set global shift functional global.vi", "Boolean 3"=FALSE}, {"Boolean"=FALSE, "Boolean 2"=FALSE, "Name"="Does custom data key exist", "Boolean 3"=FALSE}, {"Boolean"=FALSE, "Boolean 2"=FALSE, "Name"="SO Beam expander.lvlib:Read Positions.vi", "Boolean 3"=FALSE}, {"Boolean"=FALSE, "Boolean 2"=FALSE, "Name"="HHMI - Microns per Volt.vi", "Boolean 3"=FALSE}, {"Boolean"=FALSE, "Boolean 2"=FALSE, "Name"="Destroy Message handler.vi", "Boolean 3"=FALSE}, {"Boolean"=FALSE, "Boolean 2"=FALSE, "Name"="32 bit tiff reader.lvlib:Bytes to long word.vi", "Boolean 3"=FALSE}, {"Boolean"=FALSE, "Boolean 2"=FALSE, "Name"="Strip filename base and extension.vi", "Boolean 3"=FALSE}, {"Boolean"=FALSE, "Boolean 2"=FALSE, "Name"="HHMI - Define Steps for slow axis.vi", "Boolean 3"=FALSE}, {"Boolean"=FALSE, "Boolean 2"=FALSE, "Name"="HHMI - Copy finished images to UI loop display buffers.vi", "Boolean 3"=FALSE}, {"Boolean"=FALSE, "Boolean 2"=FALSE, "Name"="HHMI - Turn on just center subregion.vi", "Boolean 3"=FALSE}, {"Boolean"=FALSE, "Boolean 2"=FALSE, "Name"="HHMI - Convert between phase and grey levels.vi", "Boolean 3"=FALSE}, {"Boolean"=FALSE, "Boolean 2"=FALSE, "Name"="HHMI - Enable disable depending on scan state.vi", "Boolean 3"=FALSE}, {"Boolean"=FALSE, "Boolean 2"=FALSE, "Name"="HHMI - Calculate Signal vs Phase Function.vi", "Boolean 3"=FALSE}, {"Boolean"=FALSE, "Boolean 2"=FALSE, "Name"="HHMI - Convert Phase Ref control.vi", "Boolean 3"=FALSE}, {"Boolean"=FALSE, "Boolean 2"=FALSE, "Name"="HHMI - Is image empty.vi", "Boolean 3"=FALSE}, {"Boolean"=FALSE, "Boolean 2"=FALSE, "Name"="HHMI - Generate Integrator 1 Line.vi", "Boolean 3"=FALSE}, {"Boolean"=FALSE, "Boolean 2"=FALSE, "Name"="Search and find indices of all matches.vi", "Boolean 3"=FALSE}, {"Boolean"=FALSE, "Boolean 2"=FALSE, "Name"="su10x Reset.vi", "Boolean 3"=FALSE}, {"Boolean"=FALSE, "Boolean 2"=FALSE, "Name"="HHMI - Phase offset optimization technique functional global.vi", "Boolean 3"=FALSE}, {"Boolean"=FALSE, "Boolean 2"=FALSE, "Name"="HHMI - Convert um array to voltage array.vi", "Boolean 3"=FALSE}, {"Boolean"=FALSE, "Boolean 2"=FALSE, "Name"="String with ASCII code conversion.vi", "Boolean 3"=FALSE}, {"Boolean"=FALSE, "Boolean 2"=FALSE, "Name"="HHMI - Scale Coeffs to units of 2pi.vi", "Boolean 3"=FALSE}, {"Boolean"=FALSE, "Boolean 2"=FALSE, "Name"="Reshape 2D array to 1D XY cluster.vi", "Boolean 3"=FALSE}, {"Boolean"=FALSE, "Boolean 2"=FALSE, "Name"="HHMI - Unwrap one subregion.vi", "Boolean 3"=FALSE}, {"Boolean"=FALSE, "Boolean 2"=FALSE, "Name"="HHMI - Add current analysis image to new row in Analysis Table.vi", "Boolean 3"=FALSE}, {"Boolean"=FALSE, "Boolean 2"=FALSE, "Name"="Send Message to ENGINE.vi", "Boolean 3"=FALSE}, {"Boolean"=FALSE, "Boolean 2"=FALSE, "Name"="HHMI - Replacement type for rejected phase offset subregions functional global.vi", "Boolean 3"=FALSE}, {"Boolean"=FALSE, "Boolean 2"=FALSE, "Name"="Send Message to GUI.vi", "Boolean 3"=FALSE}, {"Boolean"=FALSE, "Boolean 2"=FALSE, "Name"="HHMI - Is SLM initialized.vi", "Boolean 3"=FALSE}, {"Boolean"=FALSE, "Boolean 2"=FALSE, "Name"="Galil CLOSE.VI", "Boolean 3"=FALSE}, {"Boolean"=FALSE, "Boolean 2"=FALSE, "Name"="HHMI - Limits at which power should be reduced.vi", "Boolean 3"=FALSE}, {"Boolean"=FALSE, "Boolean 2"=FALSE, "Name"="HHMI - Enough signal thresholds during AO scan.vi", "Boolean 3"=FALSE}, {"Boolean"=FALSE, "Boolean 2"=FALSE, "Name"="HHMI - Analysis Table column headers.vi", "Boolean 3"=FALSE}, {"Boolean"=FALSE, "Boolean 2"=FALSE, "Name"="HHMI - Convert circle Coordinates to bounding box.vi", "Boolean 3"=FALSE}, {"Boolean"=FALSE, "Boolean 2"=FALSE, "Name"="HHMI - Subregions to optimize with neighbors storage functional global.vi", "Boolean 3"=FALSE}, {"Boolean"=FALSE, "Boolean 2"=FALSE, "Name"="HHMI - Invalid COM subregion storage functional global.vi", "Boolean 3"=FALSE}, {"Boolean"=FALSE, "Boolean 2"=FALSE, "Name"="UCluClu Error Append Call Chain source first.vi", "Boolean 3"=FALSE}, {"Boolean"=FALSE, "Boolean 2"=FALSE, "Name"="#24.vi", "Boolean 3"=FALSE}, {"Boolean"=FALSE, "Boolean 2"=FALSE, "Name"="HHMI - Add time to filename base.vi", "Boolean 3"=FALSE}, {"Boolean"=FALSE, "Boolean 2"=FALSE, "Name"="HHMI - Image metadata key names.vi", "Boolean 3"=FALSE}, {"Boolean"=FALSE, "Boolean 2"=FALSE, "Name"="HHMI - AO beam reducer moved in for tilt optimization.vi", "Boolean 3"=FALSE}, {"Boolean"=FALSE, "Boolean 2"=FALSE, "Name"="HHMI - SubSub region number of rows and columns functional global.vi", "Boolean 3"=FALSE}, {"Boolean"=FALSE, "Boolean 2"=FALSE, "Name"="HHMI - Clicked XY coordinate functional global.vi", "Boolean 3"=FALSE}, {"Boolean"=FALSE, "Boolean 2"=FALSE, "Name"="INI Create Semaphore.vi", "Boolean 3"=FALSE}, {"Boolean"=FALSE, "Boolean 2"=FALSE, "Name"="Time since T0.vi", "Boolean 3"=FALSE}, {"Boolean"=FALSE, "Boolean 2"=FALSE, "Name"="HHMI - Signal window Preferences.vi", "Boolean 3"=FALSE}, {"Boolean"=FALSE, "Boolean 2"=FALSE, "Name"="Initialize Message handler.vi", "Boolean 3"=FALSE}, {"Boolean"=FALSE, "Boolean 2"=FALSE, "Name"="HHMI - Subregion scan type functional global.vi", "Boolean 3"=FALSE}, {"Boolean"=FALSE, "Boolean 2"=FALSE, "Name"="HHMI - Number of Slow axis points in Ramp waveform.vi", "Boolean 3"=FALSE}, {"Boolean"=FALSE, "Boolean 2"=FALSE, "Name"="HHMI - Cal Zernike Angular part.vi", "Boolean 3"=FALSE}, {"Boolean"=FALSE, "Boolean 2"=FALSE, "Name"="HHMI - AO steps to optimize functional global.vi", "Boolean 3"=FALSE}, {"Boolean"=FALSE, "Boolean 2"=FALSE, "Name"="32 bit tiff reader.lvlib:Bytes to word.vi", "Boolean 3"=FALSE}, {"Boolean"=FALSE, "Boolean 2"=FALSE, "Name"="HHMI - Convert pixels to microns.vi", "Boolean 3"=FALSE}, {"Boolean"=FALSE, "Boolean 2"=FALSE, "Name"="Return space.vi", "Boolean 3"=FALSE}, {"Boolean"=FALSE, "Boolean 2"=FALSE, "Name"="HHMI - Check if Signal is too low.vi", "Boolean 3"=FALSE}, {"Boolean"=FALSE, "Boolean 2"=FALSE, "Name"="Reshape 2D array to 1D I32.vi", "Boolean 3"=FALSE}, {"Boolean"=FALSE, "Boolean 2"=FALSE, "Name"="Reshape 2D array to 1D I16.vi", "Boolean 3"=FALSE}, {"Boolean"=FALSE, "Boolean 2"=FALSE, "Name"="Reshape 2D array to 1D DBL.vi", "Boolean 3"=FALSE}, {"Boolean"=FALSE, "Boolean 2"=FALSE, "Name"="HHMI - Ramp array sizes.vi", "Boolean 3"=FALSE}, {"Boolean"=FALSE, "Boolean 2"=FALSE, "Name"="Reshape 2D array to 1D Bool.vi", "Boolean 3"=FALSE}, {"Boolean"=FALSE, "Boolean 2"=FALSE, "Name"="Reshape 2D array to 1D SGL.vi", "Boolean 3"=FALSE}, {"Boolean"=FALSE, "Boolean 2"=FALSE, "Name"="Get last column.vi", "Boolean 3"=FALSE}, {"Boolean"=FALSE, "Boolean 2"=FALSE, "Name"="Strip N levels off path.vi", "Boolean 3"=FALSE}, {"Boolean"=FALSE, "Boolean 2"=FALSE, "Name"="Generate Sinc.vi", "Boolean 3"=FALSE}, {"Boolean"=FALSE, "Boolean 2"=FALSE, "Name"="HHMI - Center subregion index.vi", "Boolean 3"=FALSE}, {"Boolean"=FALSE, "Boolean 2"=FALSE, "Name"="HHMI - Beam size where beam reducer is used.vi", "Boolean 3"=FALSE}, {"Boolean"=FALSE, "Boolean 2"=FALSE, "Name"="2D Mean.vi", "Boolean 3"=FALSE}, {"Boolean"=FALSE, "Boolean 2"=FALSE, "Name"="HHMI - Calc X wave for ramp.vi", "Boolean 3"=FALSE}, {"Boolean"=FALSE, "Boolean 2"=FALSE, "Name"="su10x Close.vi", "Boolean 3"=FALSE}, {"Boolean"=FALSE, "Boolean 2"=FALSE, "Name"="HHMI - Convert Find Image Shift control.vi", "Boolean 3"=FALSE}, {"Boolean"=FALSE, "Boolean 2"=FALSE, "Name"="HHMI - Reference subregion functional global.vi", "Boolean 3"=FALSE}, {"Boolean"=FALSE, "Boolean 2"=FALSE, "Name"="HHMI - Locate blob algorithm f global.vi", "Boolean 3"=FALSE}, {"Boolean"=FALSE, "Boolean 2"=FALSE, "Name"="HHMI - Phase reference type during AO scan.vi", "Boolean 3"=FALSE}, {"Boolean"=FALSE, "Boolean 2"=FALSE, "Name"="HHMI - Phase magnification functional global.vi", "Boolean 3"=FALSE}, {"Boolean"=FALSE, "Boolean 2"=FALSE, "Name"="HHMI - X or Y or Z Parameters to origin coords.vi", "Boolean 3"=FALSE}, {"Boolean"=FALSE, "Boolean 2"=FALSE, "Name"="HHMI - Reject percentage threshold during optimization functional global.vi", "Boolean 3"=FALSE}, {"Boolean"=FALSE, "Boolean 2"=FALSE, "Name"="HHMI - Check Window Bounds.vi", "Boolean 3"=FALSE}, {"Boolean"=FALSE, "Boolean 2"=FALSE, "Name"="HHMI - Pockel cell threshold functional global.vi", "Boolean 3"=FALSE}, {"Boolean"=FALSE, "Boolean 2"=FALSE, "Name"="HHMI - Number of angle adjustment iterations during AO scan.vi", "Boolean 3"=FALSE}, {"Boolean"=FALSE, "Boolean 2"=FALSE, "Name"="HHMI - Move beam reducer during AO scan.vi", "Boolean 3"=FALSE}, {"Boolean"=FALSE, "Boolean 2"=FALSE, "Name"="HHMI - Filter to power reduction.vi", "Boolean 3"=FALSE}, {"Boolean"=FALSE, "Boolean 2"=FALSE, "Name"="HHMI - Generate Integrator Pulse train.vi", "Boolean 3"=FALSE}, {"Boolean"=FALSE, "Boolean 2"=FALSE, "Name"="HHMI - Number of phase offsets to measure at for Phase match algorithm.vi", "Boolean 3"=FALSE}, {"Boolean"=FALSE, "Boolean 2"=FALSE, "Name"="HHMI - Does Zernike mode exist.vi", "Boolean 3"=FALSE}, {"Boolean"=FALSE, "Boolean 2"=FALSE, "Name"="HHMI - Convert Z um to Volts.vi", "Boolean 3"=FALSE}, {"Boolean"=FALSE, "Boolean 2"=FALSE, "Name"="HHMI - Generate Pockel.vi", "Boolean 3"=FALSE}, {"Boolean"=FALSE, "Boolean 2"=FALSE, "Name"="HHMI - Laser limits.vi", "Boolean 3"=FALSE}, {"Boolean"=FALSE, "Boolean 2"=FALSE, "Name"="HHMI - Convert Image Correlation Ref control.vi", "Boolean 3"=FALSE}, {"Boolean"=FALSE, "Boolean 2"=FALSE, "Name"="SO Beam expander.lvlib:mm to counts.vi", "Boolean 3"=FALSE}, {"Boolean"=FALSE, "Boolean 2"=FALSE, "Name"="SO Beam expander.lvlib:counts to mm.vi", "Boolean 3"=FALSE}, {"Boolean"=FALSE, "Boolean 2"=FALSE, "Name"="Append to filename base.vi", "Boolean 3"=FALSE}, {"Boolean"=FALSE, "Boolean 2"=FALSE, "Name"="HHMI - PI System Numbers.vi", "Boolean 3"=FALSE}, {"Boolean"=FALSE, "Boolean 2"=FALSE, "Name"="Get all axes.vi", "Boolean 3"=FALSE}, {"Boolean"=FALSE, "Boolean 2"=FALSE, "Name"="HHMI - Use normal circle size to determine signal global.vi", "Boolean 3"=FALSE}, {"Boolean"=FALSE, "Boolean 2"=FALSE, "Name"="HHMI - Subregion row, column to index.vi", "Boolean 3"=FALSE}, {"Boolean"=FALSE, "Boolean 2"=FALSE, "Name"="Round to nearest.vi", "Boolean 3"=FALSE}, {"Boolean"=FALSE, "Boolean 2"=FALSE, "Name"="HHMI - Subregion index to row, column.vi", "Boolean 3"=FALSE}, {"Boolean"=FALSE, "Boolean 2"=FALSE, "Name"="HHMI - XY table max speed.vi", "Boolean 3"=FALSE}, {"Boolean"=FALSE, "Boolean 2"=FALSE, "Name"="HHMI - Max seconds a 20 MHz, 24-bit timer can count.vi", "Boolean 3"=FALSE}, {"Boolean"=FALSE, "Boolean 2"=FALSE, "Name"="HHMI - Microscope objective focal length.vi", "Boolean 3"=FALSE}, {"Boolean"=FALSE, "Boolean 2"=FALSE, "Name"="HHMI - PI Ultrasonic limits (mm).vi", "Boolean 3"=FALSE}, {"Boolean"=FALSE, "Boolean 2"=FALSE, "Name"="HHMI - Z Piezo voltage limits.vi", "Boolean 3"=FALSE}, {"Boolean"=FALSE, "Boolean 2"=FALSE, "Name"="HHMI - Galvo voltage limits.vi", "Boolean 3"=FALSE}, {"Boolean"=FALSE, "Boolean 2"=FALSE, "Name"="HHMI - DAQ AI XY Position Voltage Span constant.vi", "Boolean 3"=FALSE}, {"Boolean"=FALSE, "Boolean 2"=FALSE, "Name"="HHMI - Memory conservation need above this number of pixels.vi", "Boolean 3"=FALSE}, {"Boolean"=FALSE, "Boolean 2"=FALSE, "Name"="32 bit tiff reader.lvlib:U16ToType.vi", "Boolean 3"=FALSE}, {"Boolean"=FALSE, "Boolean 2"=FALSE, "Name"="HHMI - DAQ Voltage Span constant.vi", "Boolean 3"=FALSE}, {"Boolean"=FALSE, "Boolean 2"=FALSE, "Name"="HHMI - SLM pixel size.vi", "Boolean 3"=FALSE}, {"Boolean"=FALSE, "Boolean 2"=FALSE, "Name"="HHMI - Galvo amplifier gain.vi", "Boolean 3"=FALSE}, {"Boolean"=FALSE, "Boolean 2"=FALSE, "Name"="HHMI - Voltage Low Threshold.vi", "Boolean 3"=FALSE}, {"Boolean"=FALSE, "Boolean 2"=FALSE, "Name"="HHMI - Border Size constant.vi", "Boolean 3"=FALSE}, {"Boolean"=FALSE, "Boolean 2"=FALSE, "Name"="HHMI - Max AO Rate.vi", "Boolean 3"=FALSE}, {"Boolean"=FALSE, "Boolean 2"=FALSE, "Name"="HHMI - Power increase or decrease base factor.vi", "Boolean 3"=FALSE}, {"Boolean"=FALSE, "Boolean 2"=FALSE, "Name"="HHMI - SLM added file image name to save with.vi", "Boolean 3"=FALSE}, {"Boolean"=FALSE, "Boolean 2"=FALSE, "Name"="MISSING CODE PLACEHOLDER.vi", "Boolean 3"=FALSE}]
  out "Total # standard .vis":i32=804
  # "Debug?"
  # "Reentrant?"
  # "Is Clone?"
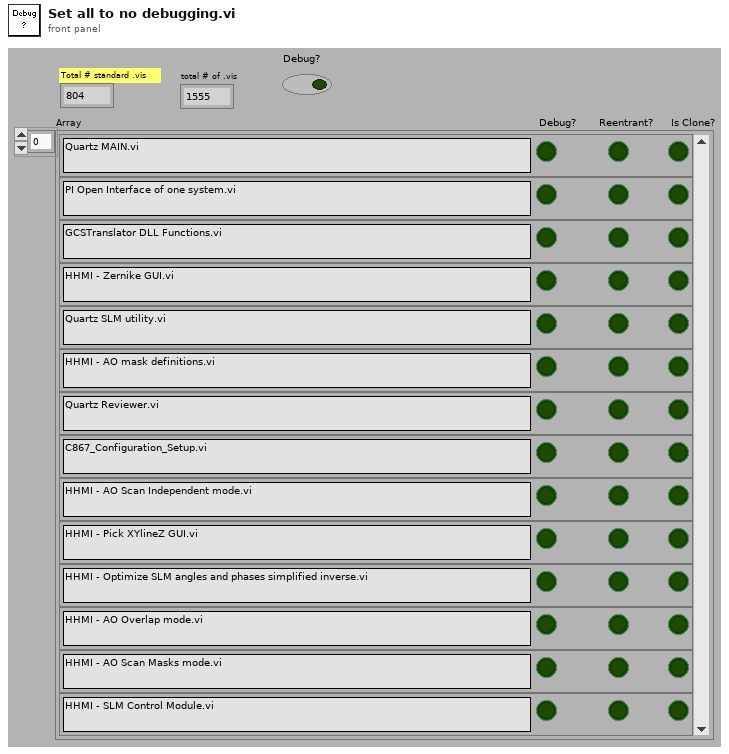
[diagram p1: front panel]
types:
  T1 = cluster{"Boolean":bool, "Boolean 2":bool, "Name":string, "Boolean 3":bool}[]
  T2 = enum32{"invalid VI type", "Standard VI", "Control VI", "Global VI", "Polymorphic VI", "Configuration VI", "SubSystem", "Facade VI", "Method VI", "Statechart Diagram VI"}
  T3 = cluster{"Path":path, "Name":string, "Exec.AllowDebug":bool, "Exec.IsReentrant":bool, "IsCloneVI":bool}
  T4 = cluster{"Path":path, "Name":string, "Exec.AllowDebug":bool, "Exec.IsReentrant":bool, "IsCloneVI":bool}[]
  T5 = cluster{"Boolean":bool, "Boolean 2":bool, "Name":string, "Boolean 3":bool}
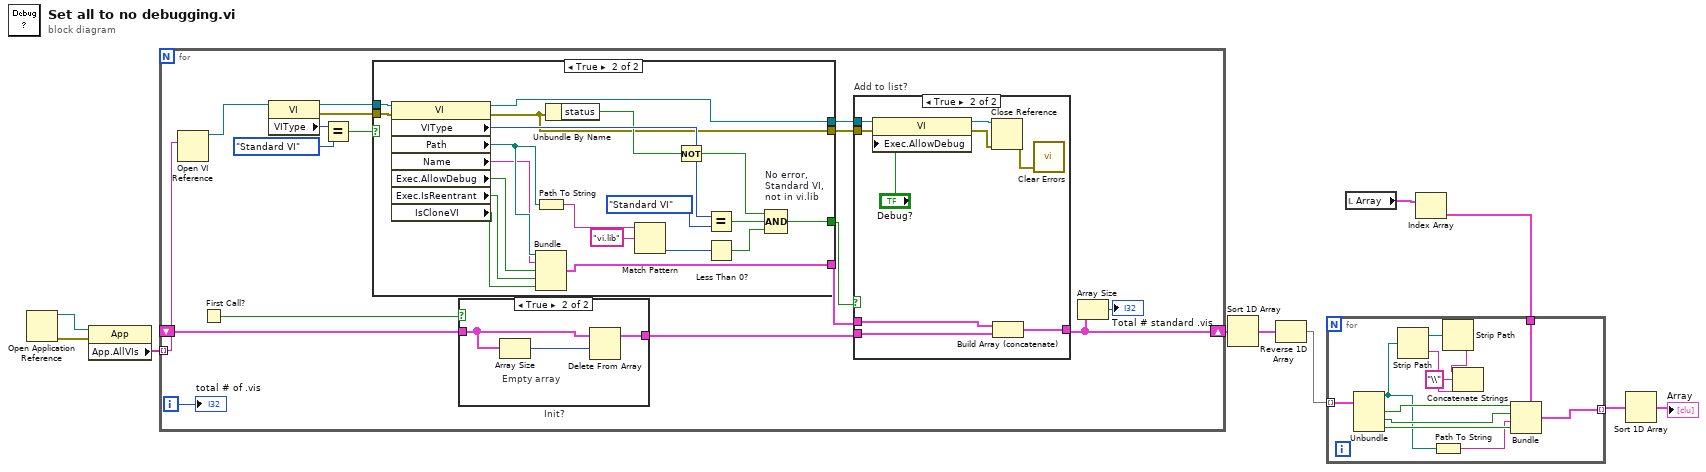
[diagram p0: block diagram]
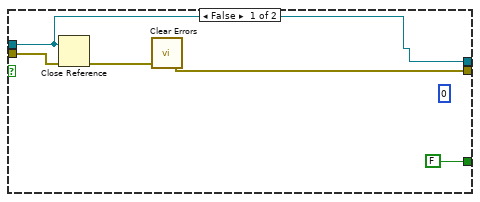
[diagram p2: hidden frame]
diagram:
  n1 = Open Application Reference() -> (0:w6:errorcluster, 3:w10:refnum<vi>)  [unwired: 1 in, 3 out]
  n2 = property class="App"(reference=w10, error in=w6) -> ("App.AllVIs"=w9:string[])  [unwired: 2 out]
  n3 = for {
    tunnel: w9 -> [w27] mode=indexing
    shift-right: [w19] -> w8
    shift-left: _ -> [w25]
    i -> [w21]
    n4 = Open VI Reference(vi path=w27) -> (vi reference=w18:refnum<vi>)  [unwired: 1 in, 5 out]
    n5 = First Call?() -> (First Call?: T/F=w23:bool)
    n6 = property class="VI"(reference=w18) -> (reference out=w17:refnum<vi>, error out=w16:errorcluster, "VIType"=w14:T2)  [unwired: 1 in]
    n7 = Equal?(x=w14, y=T2."Standard VI" ("VI Type")) -> (x = y?=w13:bool)
    n8 = case shown="True" w13 {
      tunnel: [_ w44] -> w26
      tunnel: [FALSE w43] -> w22
      tunnel: w17 -> [w28 w38]
      tunnel: w16 -> [w31 w37]
      tunnel: [w28 w36] -> w12
      tunnel: [w29 w35] -> w11
      frame False {
        (unwired) u32 0
        n9 = Close Reference(reference=w28, error in (no error)=w31) -> (error out=w30:errorcluster)
        n10 = call <vilib>:"Clear Errors.vi"("error in (no error)"=w30) -> ("error out"=w29:errorcluster)  [unwired: 6 out]
      }
      frame True {
        n11 = property class="VI"(reference=w38, error in=w37) -> (reference out=w36:refnum<vi>, error out=w35:errorcluster, "VIType"=w52:T2, "Path"=w46:path, "Name"=w45:string, "Exec.AllowDebug"=w39:bool, "Exec.IsReentrant"=w34:bool, "IsCloneVI"=w33:bool)
        n12 = Path To String(path=w46) -> (string=w47:string)
        n13 = Bundle("Path"=w46, "Name"=w45, "Exec.AllowDebug"=w39, "Exec.IsReentrant"=w34, "IsCloneVI"=w33) -> (w44:T3)  [unwired: 1 out]
        n14 = Unbundle By Name(w35) -> ("status"=w41:bool)
        n15 = Match Pattern(string=w47, regular expression="vi.lib") -> (offset past match=w49:i32)  [unwired: 4 out]
        n16 = Not(x=w41) -> (.not. x?=w40:bool)
        n17 = Equal?(x=w52, y=T2."Standard VI" ("VI Type")) -> (x = y?=w42:bool)
        n18 = Less Than 0?(x=w49) -> (x < 0?=w48:bool)
        n19 = Compound Arithmetic op=AND "No error,\nStandard VI,\nnot in vi.lib"(w40, w42, w48) -> (w43:bool)
      }
    }
    n20 = case "Init?" shown="True" w23 {
      tunnel: w25 -> [w53 w56]
      tunnel: [w53 w54] -> w24
      frame False {
      }
      frame True {
        # "Empty array"
        n21 = Array Size(array=w56) -> (size(s)=w55:i32)
        n22 = Delete From Array(array=w56, length=w55) -> (array with subset deleted=w54:T4)  [unwired: 1 in, 1 out]
      }
    }
    n23 = case "Add to list?" shown="True" w22 {
      tunnel: w24 -> [w57 w66]
      tunnel: [w57 w65] -> w19
      tunnel: w26 -> [_ w64]
      tunnel: w12 -> [_ w61]
      tunnel: w11 -> [_ w59]
      frame False {
      }
      frame True {
        n24 = property class="VI"(reference=w61, error in=w59, "Exec.AllowDebug"="Debug?") -> (reference out=w63:refnum<vi>, error out=w62:errorcluster)
        n25 = Close Reference(reference=w63, error in (no error)=w62) -> (error out=w60:errorcluster)
        n26 = Build Array (concatenate)(w64, w66) -> (w65:T4)
        n27 = call <vilib>:"Clear Errors.vi"("error in (no error)"=w60) -> ()  [unwired: 7 out]
      }
    }
    n28 = Array Size(array=w19) -> (size(s)=→"Total # standard .vis":i32)
    "total # of .vis" <- w21
  }
  n29 = Sort 1D Array(array=w8) -> (sorted array=w7:T4)
  n30 = Reverse 1D Array(array=w7) -> (reversed array=w5:T4)
  n31 = local read "Array"() -> (w2:T1)
  n32 = Index Array(array=w2) -> (element=w1:T5)  [unwired: 1 in]
  n33 = for {
    tunnel: w5 -> [w78] mode=indexing
    tunnel: [w77] -> w4 mode=indexing
    tunnel: w1 -> [w70]
    n34 = Unbundle(w78) -> ("Path"=w68:path, "Exec.AllowDebug"=w72:bool, "Exec.IsReentrant"=w71:bool, "IsCloneVI"=w69:bool)  [unwired: 1 out]
    n35 = Strip Path(path=w68) -> (stripped path=w76:path, name=w75:string)
    n36 = Path To String(path=w68) -> (string=w67:string)
    n37 = Strip Path(path=w76) -> (name=w74:string)  [unwired: 1 out]
    n38 = Concatenate Strings(w74, "\\" ("string"), w75) -> ()  [unwired: 1 out]
    n39 = Bundle(cluster=w70, "Boolean"=w72, "Boolean 2"=w71, "Name"=w67, "Boolean 3"=w69) -> (w77:T5)
  }
  n40 = Sort 1D Array(array=w4) -> (sorted array=→"Array":T1)
